vi "tvac_gui_chamber_workingcopy.vi"() -> ()   [LabVIEW 2017]
uses:
  <vilib>/httpClient/ClientHandle.ctl
  msg7171_linux.llb/send single message.vi
  <vilib>/httpClient/POSTBuffer.vi
  <vilib>/httpClient/LabVIEWHTTPClient.lvlib
panel:
  in  "Read MCC":bool
  in  "Read Pressure Gauges":bool
  out "output cluster":T1
  out "Cluster":T2
  in  "Custom Graph Selector":i32
  in  "exit":bool
  in  "AlarmColor":u32(colorbox)
  in  "Alarm String":string
  in  "Plot Color":u32(colorbox)=16860
  in  "Temperature":dbl format="%#_13g"
  in  "TC Label":string
  in  "Graph ON/OFF":u32(colorbox)=4250624
  in  "index (col)":i32
  in  "index (row)":i32
  out "working array":bool[](array[boolean])
  in  "Local Debug":bool
  in  "Tab Control":enum32{"TCs", "Graphs", "Thermal Profile"}(tab)
  in  "Log/Linear Y-Axis":u16(ring) items=["Linear", "Log"]
  in  "Total Time":dbl
  in  "Set Time TC Graph":bool
  in  "Graphing Selection":u16(ring) items=["User Selection", "Graph All Thermocouples", "Clear Graph"]
  in  "Time Scale":u16(ring) items=["Minutes", "Hours", "Seconds"]
  out "Waveform Chart":waveform(dbl)[](graph)
  out "Thermocouples":T3(array[cluster])
  in  "Log/Linear Y-Axis 6":u16(ring) items=["Linear", "Log"]
  in  "Log/Linear Y-Axis 5":u16(ring) items=["Linear", "Log"]
  in  "Log/Linear Y-Axis 3":u16(ring) items=["Linear", "Log"]
  in  "Log/Linear Y-Axis 2":u16(ring) items=["Linear", "Log"]
  in  "Total Time 6":dbl
  in  "Set Time TC Graph 6":bool
  in  "Time Scale 6":u16(ring) items=["Minutes", "Hours", "Seconds"]
  in  "Total Time 5":dbl
  in  "Set Time TC Graph 5":bool
  in  "Time Scale 5":u16(ring) items=["Minutes", "Hours", "Seconds"]
  in  "Total Time 4":dbl
  in  "Set Time TC Graph 4":bool
  in  "Time Scale 4":u16(ring) items=["Minutes", "Hours", "Seconds"]
  in  "Total Time 3":dbl
  in  "Set Time TC Graph 3":bool
  in  "Time Scale 3":u16(ring) items=["Minutes", "Hours", "Seconds"]
  in  "Total Time 2":dbl
  in  "Set Time TC Graph 2":bool
  in  "Time Scale 2":u16(ring) items=["Minutes", "Hours", "Seconds"]
  in  "Log/Linear Y-Axis 1":u16(ring) items=["Linear", "Log"]
  in  "Total Time 1":dbl
  in  "Set Time TC Graph 1":bool
  in  "Time Scale 1":u16(ring) items=["Minutes", "Hours", "Seconds"]
  in  "Custom Chart 2 Selection":i32[](listbox)=[0]
  in  "Custom Chart 1 Selection":i32[](listbox)=[0]
  out "Custom Chart 1":waveform(dbl)[](graph)
  in  "Custom Chart 3 Selection":i32[](listbox)=[0]
  in  "Custom Chart 4 Selection":i32[](listbox)=[0]
  in  "Custom Chart 5 Selection":i32[](listbox)=[0]
  in  "Custom Chart 6 Selection":i32[](listbox)=[0]
  out "Custom Chart 2":waveform(dbl)[](graph)
  out "Custom Chart 3":waveform(dbl)[](graph)
  out "Custom Chart 4":waveform(dbl)[](graph)
  out "Custom Chart 5":waveform(dbl)[](graph)
  out "Custom Chart 6":waveform(dbl)[](graph)
  in  "Log/Linear Y-Axis 4":u16(ring) items=["Linear", "Log"]
  in  "Set Z 1":bool
  in  "Z3 Thermal Profile":i32(listbox)
  in  "Z2 Thermal Profile":i32(listbox)
  in  "Z1 Thermal Profile":i32(listbox)
  in  "Zone 3 Temp":u16(ring) items=["Average", "Minimum", "Maximum"]
  in  "Zone 2 Temp":u16(ring) items=["Average", "Minimum", "Maximum"]
  in  "Zone 1 Temp":u16(ring) items=["Average", "Minimum", "Maximum"]
  in  "Zone 1 TC":i32[](listbox)=[0]
  in  "Zone 2 TC":i32[](listbox)=[0]
  in  "Zone 3 TC":i32[](listbox)=[0]
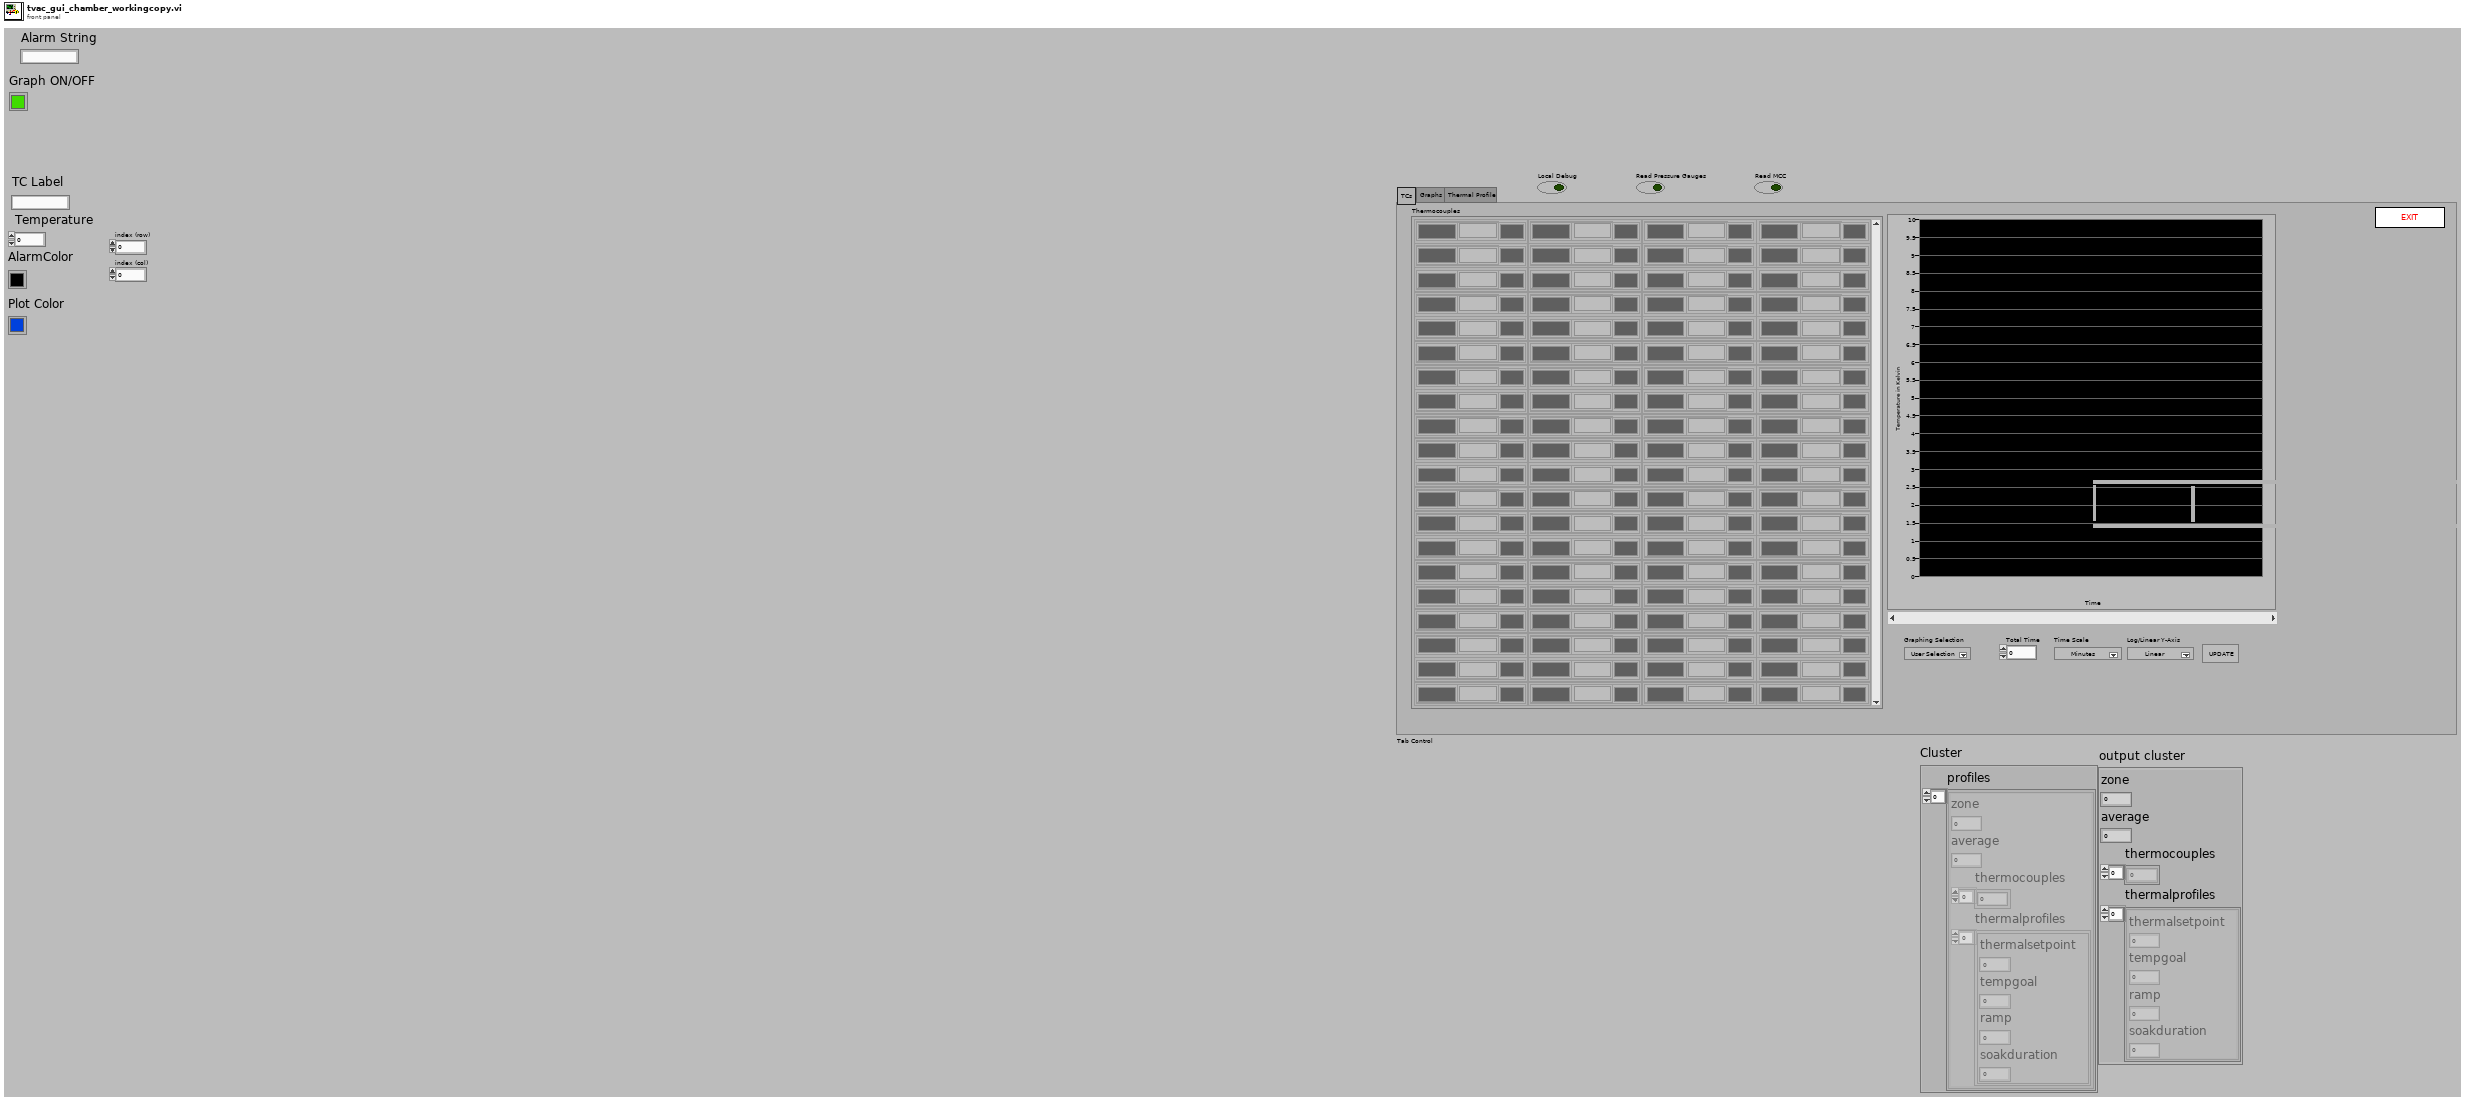
[diagram p1: front panel]
types:
  T1 = cluster{"zone":i32, "average":i32, "thermocouples":dbl[], "thermalprofiles":cluster{"thermalsetpoint":i32, "tempgoal":i32, "ramp":i32, "soakduration":i32}[]}
  T2 = cluster{"profiles":cluster{"zone":i32, "average":i32, "thermocouples":dbl[], "thermalprofiles":cluster{"thermalsetpoint":i32, "tempgoal":i32, "ramp":i32, "soakduration":i32}[]}[]}
  T3 = cluster{"TC Label":string, "Alarm Status":string, "Alarm Color":u32, "Temperature":string, "PlotColor":u32, "Graph On/Off":u32}[][]
  T4 = cluster{"Cp Stage 1 Temp":dbl[], "Cp Stage 2 Temp":dbl[], "Compressor Temp":dbl[]}
  T5 = typedef "LabVIEWHTTPClient.lvlib/ClientHandle.ctl" = refnum<k1>
  T6 = cluster{"go":bool, "Http session":T5, "URL prefex":string, "index (row)":i32, "index (col)":i32, "Graph ON/OFF":u32, "TC Label":string, "Temperature":dbl, "AlarmColor":u32, "Plot Color":u32, "Alarm String":string, "Thermocouples":cluster{"TC Label":string, "Alarm Status":string, "Alarm Color":u32, "Temperature":string, "PlotColor":u32, "Graph On/Off":u32}[][], "working array":bool[], "i":i32, "NumberTCs":i32, "Waveform Chart":waveform(dbl)[], "Custom Chart 1":waveform(dbl)[], "Pressure":dbl[], "numSensors":i32, "Database":dbl[], "PumpTemps":cluster{"Cp Stage 1 Temp":dbl[], "Cp Stage 2 Temp":dbl[], "Compressor Temp":dbl[]}, "Zones":dbl[]}
  T7 = cluster{"TC Label":string, "Alarm Status":string, "Alarm Color":u32, "Temperature":string, "PlotColor":u32, "Graph On/Off":u32}
  T8 = cluster{"Cryopump Stage 1 Temp":dbl[], "Cryopump Stage 2 Temp":dbl[], "Compressor Temp":dbl[]}
  T9 = cluster{"DutyCycle":i32, "Stage1Temp":i32, "CryoPumpReadyState":cluster{"MotorOn":bool, "Ready":bool}, "PurgeValveState":bool, "RegenError":string, "RegenStep":string, "RoughingValveState":bool, "RoughingInterlock":cluster{"RoughingPermission":bool, "RoughingNeeded":bool, "Cryopumprunning":bool}, "Stage2Temp":i32, "Status":cluster{"PumpOn":bool, "RoughOpen":bool, "PurgeOpen":bool, "ThermocoupleGaugeOn":bool, "PowerFailureOccurred":bool}, "TcPressure":i32}
  T10 = cluster{"time":string, "TCs":cluster{"thermocouple":i32, "time":dbl, "temp":dbl, "working":bool, "alarm":i32}[]}
  T11 = cluster{"thermocouple":i32, "time":dbl, "temp":dbl, "working":bool, "alarm":i32}[]
  T12 = typedef "LVPositionTypeDef.ctl" = cluster{"Left":i32, "Top":i32}
  T13 = typedef "LVPoint32TypeDef.ctl" = cluster{"Horizontal":i32, "Vertical":i32}
  T14 = typedef "LVRangeTypeDef.ctl" = cluster{"Minimum":dbl, "Maximum":dbl, "Increment":dbl, "Minor Increment":dbl, "Start":dbl}
  T15 = cluster{"Pressure[0]":dbl, "Pressure[1]":dbl, "Pressure[2]":dbl}
  T16 = cluster{"zone":i32, "average":i32, "thermocouples":dbl[], "thermalprofiles":cluster{"thermalsetpoint":i32, "tempgoal":i32, "ramp":i32, "soakduration":i32}[]}[]
  T17 = cluster{"profiles[0]":cluster{"zone":i32, "average":i32, "thermocouples":dbl[], "thermalprofiles":cluster{"thermalsetpoint":i32, "tempgoal":i32, "ramp":i32, "soakduration":i32}[]}, "profiles[1]":cluster{"zone":i32, "average":i32, "thermocouples":dbl[], "thermalprofiles":cluster{"thermalsetpoint":i32, "tempgoal":i32, "ramp":i32, "soakduration":i32}[]}, "profiles[2]":cluster{"zone":i32, "average":i32, "thermocouples":dbl[], "thermalprofiles":cluster{"thermalsetpoint":i32, "tempgoal":i32, "ramp":i32, "soakduration":i32}[]}, "profiles[3]":cluster{"zone":i32, "average":i32, "thermocouples":dbl[], "thermalprofiles":cluster{"thermalsetpoint":i32, "tempgoal":i32, "ramp":i32, "soakduration":i32}[]}, "profiles[4]":cluster{"zone":i32, "average":i32, "thermocouples":dbl[], "thermalprofiles":cluster{"thermalsetpoint":i32, "tempgoal":i32, "ramp":i32, "soakduration":i32}[]}, "profiles[5]":cluster{"zone":i32, "average":i32, "thermocouples":dbl[], "thermalprofiles":cluster{"thermalsetpoint":i32, "tempgoal":i32, "ramp":i32, "soakduration":i32}[]}, "profiles[6]":cluster{"zone":i32, "average":i32, "thermocouples":dbl[], "thermalprofiles":cluster{"thermalsetpoint":i32, "tempgoal":i32, "ramp":i32, "soakduration":i32}[]}, "profiles[7]":cluster{"zone":i32, "average":i32, "thermocouples":dbl[], "thermalprofiles":cluster{"thermalsetpoint":i32, "tempgoal":i32, "ramp":i32, "soakduration":i32}[]}, "profiles[8]":cluster{"zone":i32, "average":i32, "thermocouples":dbl[], "thermalprofiles":cluster{"thermalsetpoint":i32, "tempgoal":i32, "ramp":i32, "soakduration":i32}[]}}
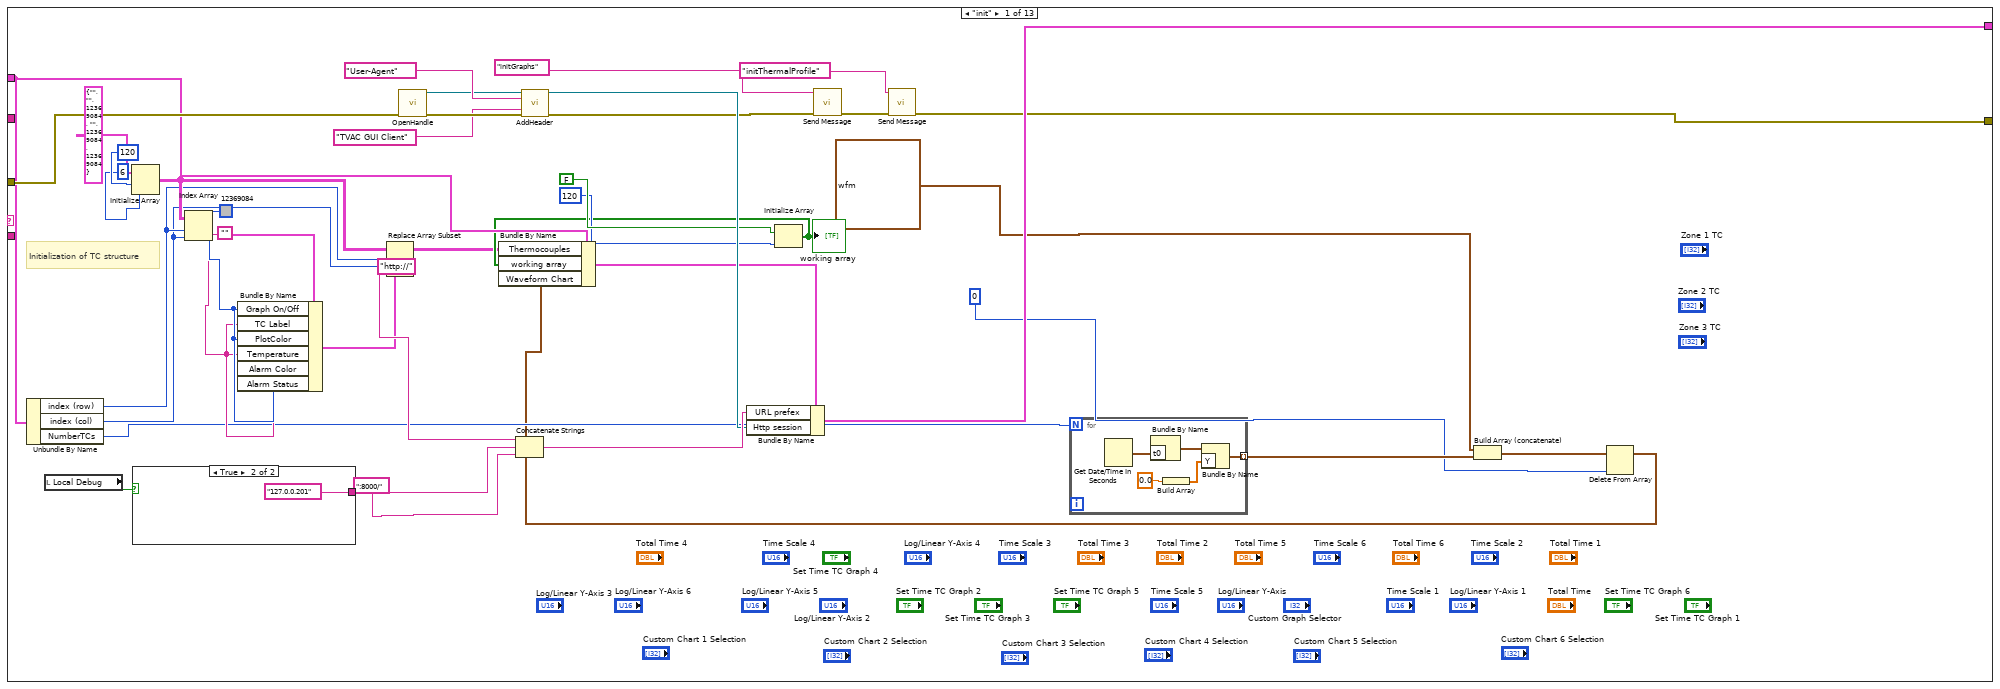
[diagram p2: hidden frame]
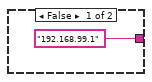
[diagram p3: hidden frame]
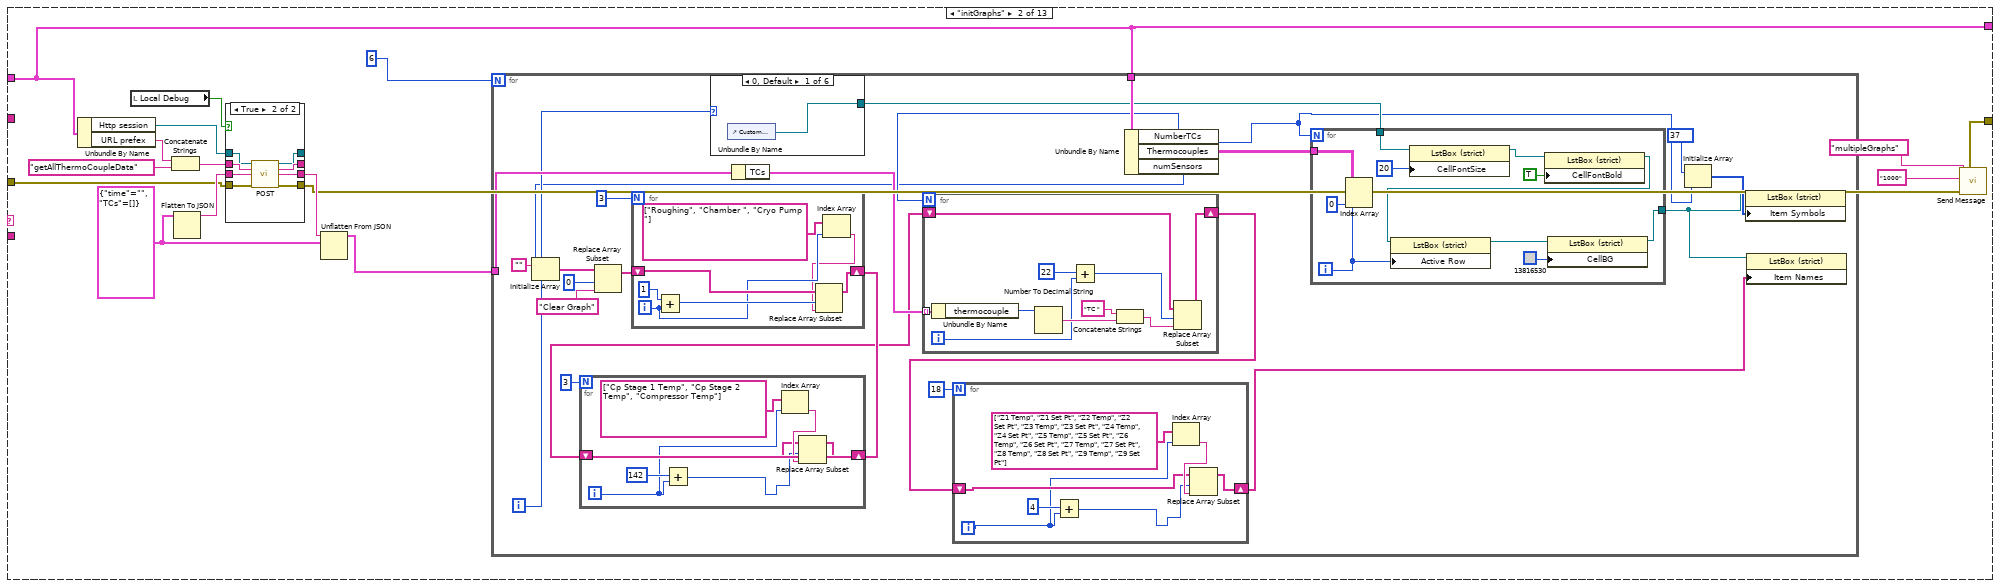
[diagram p4: hidden frame]
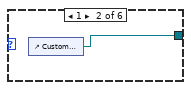
[diagram p5: hidden frame]
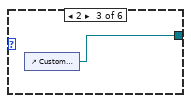
[diagram p6: hidden frame]
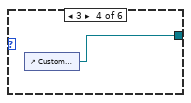
[diagram p7: hidden frame]
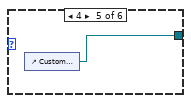
[diagram p8: hidden frame]
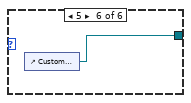
[diagram p9: hidden frame]
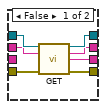
[diagram p10: hidden frame]
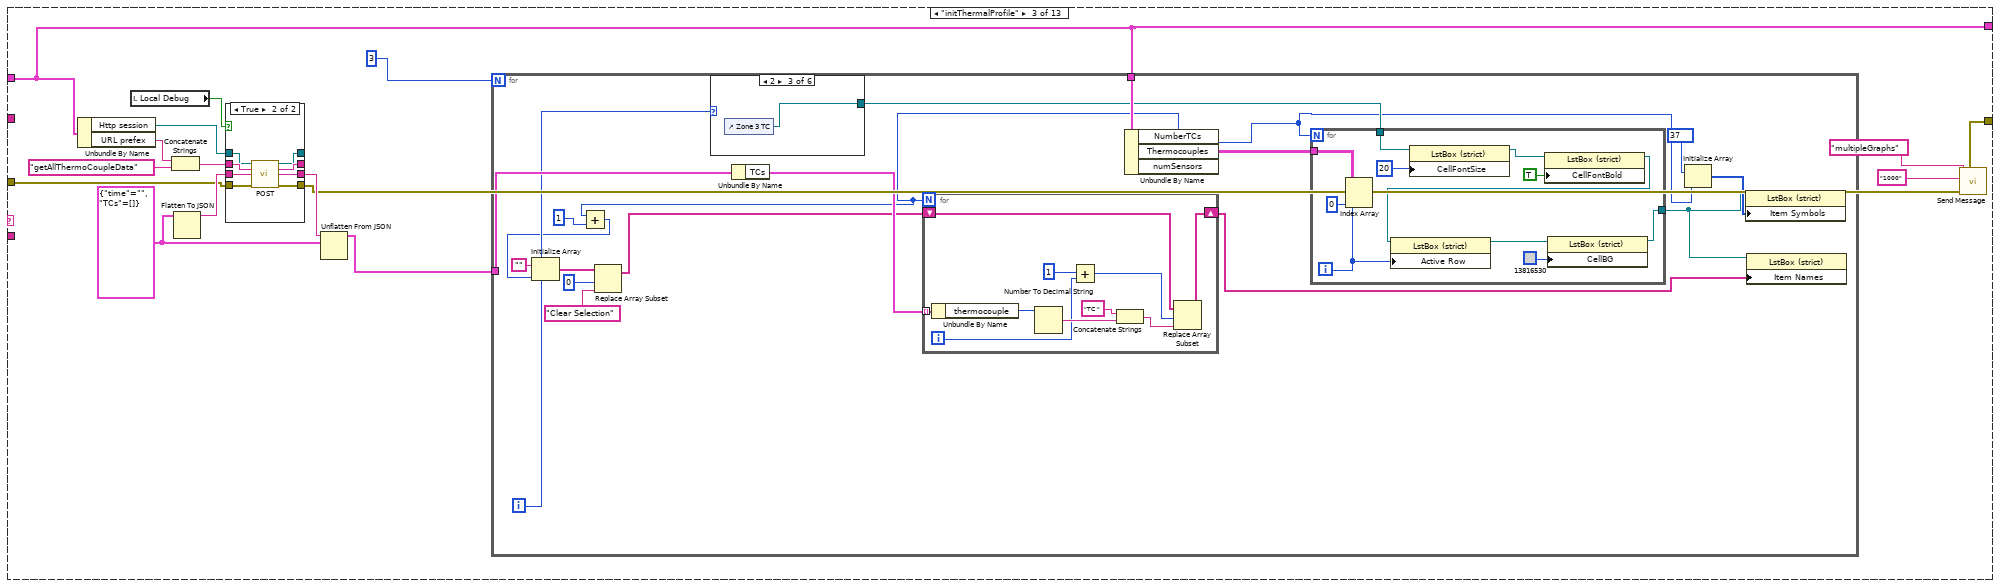
[diagram p11: hidden frame]
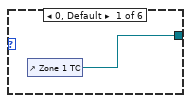
[diagram p12: hidden frame]
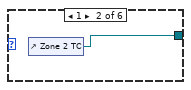
[diagram p13: hidden frame]
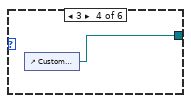
[diagram p14: hidden frame]
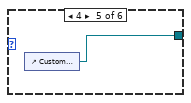
[diagram p15: hidden frame]
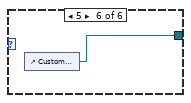
[diagram p16: hidden frame]
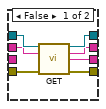
[diagram p17: hidden frame]
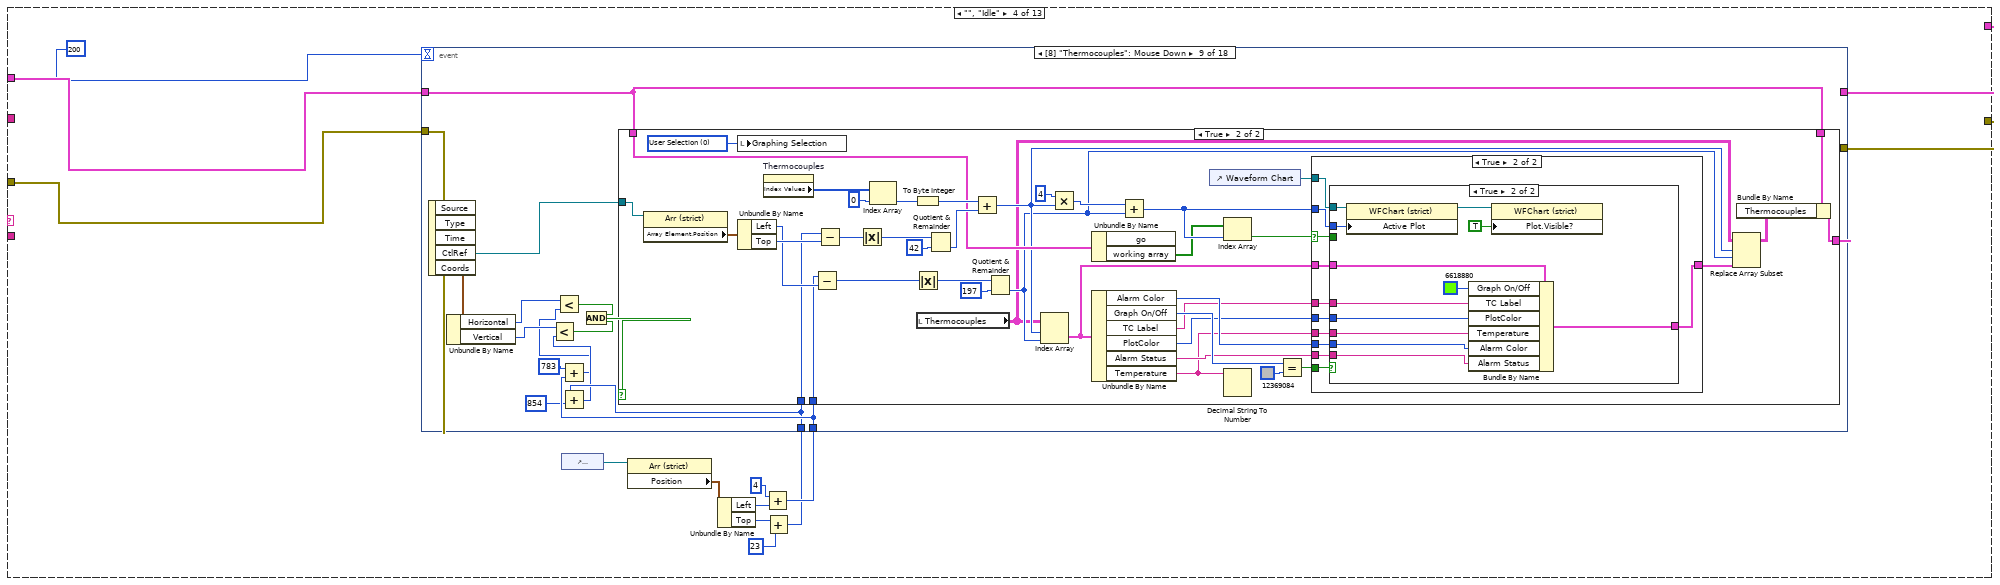
[diagram p18: hidden frame]
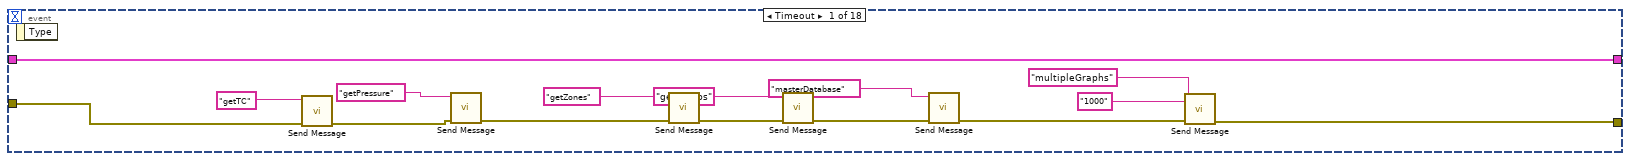
[diagram p19: hidden frame]
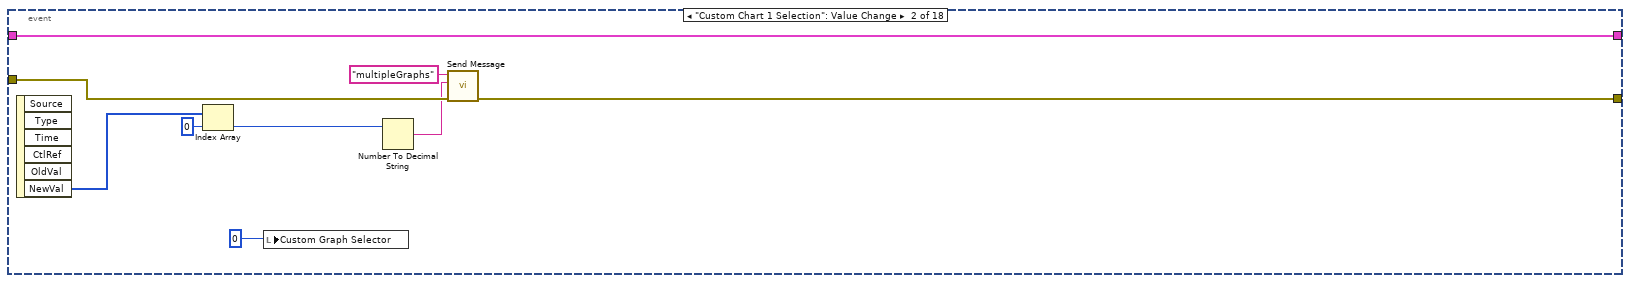
[diagram p20: hidden frame]
diagram:
  w2 = T4 {"Cp Stage 1 Temp"=[0.0], "Cp Stage 2 Temp"=[0.0], "Compressor Temp"=[0.0]}  # PumpTemps
  w5 = dbl[] []  # Pressure
  w25 = ""  # URL prefex
  w26 = T5 refnum  # Http session
  w27 = TRUE  # go
  n1 = call "Register Module.vi"() -> ("error out"=w23:errorcluster)  [unwired: 10 in, 1 out]
  n2 = call-poly "Send Message.vi"("error in (no error)"=w23, "event"="init") -> ("error out"=w22:errorcluster)  [unwired: 9 in]
  n3 = local read "Waveform Chart"() -> (w9:waveform(dbl)[])
  n4 = local read "Thermocouples"() -> (w7:T3)
  n5 = local read "Custom Chart 1"() -> (w6:waveform(dbl)[])
  n6 = Bundle("go"=w27, "Http session"=w26, "URL prefex"=w25, "index (row)"="index (row)", "index (col)"="index (col)", "Graph ON/OFF"="Graph ON/OFF", "TC Label"="TC Label", "Temperature"="Temperature", "AlarmColor"="AlarmColor", "Plot Color"="Plot Color", "Alarm String"="Alarm String", "Thermocouples"=w7, "working array"=bool[] [TRUE, TRUE, TRUE, TRUE, TRUE, TRUE, TRUE, TRUE, TRUE, TRUE, TRUE, TRUE, TRUE, TRUE, TRUE, TRUE, TRUE, TRUE, TRUE, TRUE, TRUE, TRUE, TRUE, TRUE, TRUE, TRUE, TRUE, TRUE, TRUE, TRUE, TRUE, TRUE, TRUE, TRUE, TRUE, TRUE, TRUE, TRUE, TRUE, TRUE, TRUE, TRUE, TRUE, TRUE, TRUE, TRUE, TRUE, TRUE, TRUE, TRUE, TRUE, TRUE, TRUE, TRUE, TRUE, TRUE, TRUE, TRUE, TRUE, TRUE, TRUE, TRUE, TRUE, TRUE, TRUE, TRUE, TRUE, TRUE, TRUE, TRUE, TRUE, TRUE, TRUE, TRUE, TRUE, TRUE, TRUE, TRUE, TRUE, TRUE, TRUE, TRUE, TRUE, TRUE, TRUE, TRUE, TRUE, TRUE, TRUE, TRUE, TRUE, TRUE, TRUE, TRUE, TRUE, TRUE, TRUE, TRUE, TRUE, TRUE, TRUE, TRUE, TRUE, TRUE, TRUE, TRUE, TRUE, TRUE, TRUE, TRUE, TRUE, TRUE, TRUE, TRUE, TRUE, TRUE, TRUE, TRUE, TRUE, TRUE], "i"=0, "NumberTCs"=120, "Waveform Chart"=w9, "Custom Chart 1"=w6, "Pressure"=w5, "numSensors"=145, "Database"=dbl[] [0.0, 1000.5841582194602, 1000.5841582194602, 1000.5841582194602, 0.6389895835935778, 0.7578061575842531, 1.153531014677555, 1.4572061556343079, 1.0192558642672256, 0.9245021790184325, 0.34311035179988925, 1.1970333160202968, 1.066989851322369, 0.5926593131154867, 0.7219240511326698, 1.0529790116491695, 1.4485694746891444, 0.9139060201605569, 0.7997359753068659, 0.6568795179977746, 0.8470104541419833, 1.0272585161866683, 0.6577301535824354, 0.645139941938139, 1.5235316442408067, 0.5128651184775285, 1.6421980587090137, 1.3961508335147417, 1.1242639015795428, 1.5954313466624428, 1.1919135255187876, 1.2615004458206727, 1.1320092264321664, 1.922759836270222, 1.1315561200367314, 1.4924621723754858, 0.6988771274186227, 1.069709701591943, 0.9920698240997152, 0.5395549253287656, 0.42891479657680576, 1.2794224940227927, 0.2687949632437338, 0.16127136772755854, 1.0174597006256374, 1.2079238230365172, 0.9745554383837218, 1.5348516925460962, 0.9488878852839246, 1.6634477658652282, 1.1924291951744272, 1.2231949298067308, 1.2223766746774598, 1.30664154589907, 1.2872878364107239, 0.5274250065177812, 0.7905999067114673, 1.2748974665085449, 1.216972941585413, 0.959115576325391, 0.5743502840762814, 0.8219540421676025, 0.613053899308251, 1.3785560870413707, 1.034117232127813, 1.1237698659753859, 1.4495548642149667, 0.6967905980938514, 0.6224497255665377, 1.6551326273040576, 1.2103048396824558, 0.6078721016951973, 1.3790669246280296, 0.5454332940871525, 1.5318777012492035, 1.2496539590411258, 0.9145395304446965, 1.3855381787793546, 1.0857600342029163, 1.3185833631438346, 0.9769688683142593, 1.026663691242448, 0.6744610422623843, 1.1965175398567691, 0.4847084945450119, 0.6435799980029115, 0.8079659363810663, 0.9130053929540112, 0.5271098423006861, 0.8088111736464799, 1.1455315536576556, 1.139809531926708, 1.5840192673434794, 1.0296748968089129, 1.7370669751200136, 1.3715484550405317, 0.3362063953932494, 1.0385868418202253, 1.4947740276021626, 1.0393600693910505, 0.8870410800672984, 1.2470388696569872, 0.9846724980375481, 0.9952471377109308, 1.0807485178906029, 1.1016630607035562, 1.3301039036808464, 0.8856852816151205, 0.4719509873120426, 0.5191430277856135, 0.12135113366044793, 0.4230478635224125, 1.1140562049976255, 1.5484968368781251, 1.1999891199114734, 1.8721302183420216, 1.071489235222563, 0.6260864330445979, 1.0305668002030492, 1.0223711899566386, 0.7842533472819472, 1.7301290335750898, 1.318694748426881, 0.6978662965493679], "PumpTemps"=w2, "Zones"=dbl[] [24.54828257301887, 25.0, 20.035959453954195, 26.0, 28.926820041278148, 27.0, 21.321976066931608, 28.0, 29.197600688359813, 29.0, 29.117373424110085, 30.0, 21.092914485312942, 31.0, 27.791581465649088, 32.0, 24.70861457288988, 33.0]) -> (w13:T6)  [unwired: 1 in]
  n7 = while {
    shift-left: w13 -> [w32]
    shift-right: [w29] -> _
    shift-right: [w30] -> w8
    shift-left: w22 -> [w37]
    stop <- w28 continue-if-true
    n8 = call "Get Message.vi"("error in (no error)"=w37) -> ("error out"=w35:errorcluster, "event buffer"=w36:string, "event"=w34:string, "source"=w33:string)  [unwired: 7 in]
    n9 = case shown="\"getZones\"" w34 {
      selector: w34 -> [_ _ _ _ _ _ _ _ _ _ _ _ w1352]
      tunnel: [w69 w90 w192 w273 w947 w984 w1099 w1139 w1184 w1204 w1335 w1350 w1354] -> w29
      tunnel: w32 -> [w50 w90 w192 w275 w950 w990 w1094 w1134 w1185 w1204 w1335 w1346 w1354]
      tunnel: w36 -> [_ _ _ _ _ _ _ _ _ w1205 _ _ _]
      tunnel: w35 -> [w72 w89 w191 w274 w949 w1006 w1093 w1140 w1190 _ _ w1349 w1353]
      tunnel: [w39 w85 w187 w272 w948 w980 w1093 w1140 w1190 _ _ w1348 w1351] -> w31
      tunnel: w33 -> [_ _ _ _ _ _ _ _ _ _ _ _ _]
      frame "init" {
        w55 = ""
        w56 = u32 12369084 ("PlotColor")
        # "Initialization of TC structure"
        n10 = Unbundle By Name(w50) -> ("index (row)"=w58:i32, "index (col)"=w57:i32, "NumberTCs"=w47:i32)
        n11 = local read "Local Debug"() -> (w63:bool)
        n12 = Initialize Array(T7 {"TC Label"="", "Alarm Status"="", "Alarm Color"=12369084, "Temperature"="", "PlotColor"=12369084, "Graph On/Off"=12369084}, 120 ("dimension size"), 6 ("dimension size")) -> (w59:T3)
        n13 = case shown="True" w63 {
          tunnel: ["192.168.99.1" ("Address") "127.0.0.201" ("Address")] -> w64
          frame False {
          }
          frame True {
          }
        }
        n14 = Index Array(array=w59, index (row)=w58, index (col)=w57) -> (element=w54:T7)
        n15 = Bundle By Name(cluster=w54, "Graph On/Off"=w56, "TC Label"=w55, "PlotColor"=w56, "Temperature"=w55, "Alarm Color"=w56, "Alarm Status"=w55) -> (w53:T7)
        n16 = Replace Array Subset(array=w59, new element=w53, index (row)=w58, index (col)=w57) -> (w41:T3)
        n17 = call <vilib>:"OpenHandle.vi"("error in (no error)"=w72) -> ("client handle out"=w73:T5, "error out"=w76:errorcluster)  [unwired: 13 in]
        n18 = Concatenate Strings("http://" ("url"), w64, ":8000/" ("url")) -> (w68:string)
        n19 = call <vilib>:"AddHeader.vi"("client handle"=w73, "header"="User-Agent", "value"="TVAC GUI Client", "error in (no error)"=w76) -> ("client handle out"=w67:T5, "error out"=w66:errorcluster)  [unwired: 10 in]
        n20 = Initialize Array(FALSE ("Boolean"), 120 ("dimension size")) -> (w48:bool[])
        "working array" <- w48
        n21 = call-poly "Send Message.vi"("error in (no error)"=w66, "event"="initGraphs") -> ("error out"=w40:errorcluster)  [unwired: 9 in]
        n22 = call-poly "Send Message.vi"("error in (no error)"=w40, "event"="initThermalProfile") -> ("error out"=w39:errorcluster)  [unwired: 9 in]
        n23 = for {
          N: w47 -> [_]
          tunnel: [w77] -> w45 mode=indexing
          n24 = Get Date/Time In Seconds() -> (seconds since 1Jan1904=w81:timestamp)
          n25 = Bundle By Name("t0"=w81) -> (w78:waveform(dbl))  [unwired: 1 in]
          n26 = Build Array(0.0) -> (w80:dbl[])
          n27 = Bundle By Name(cluster=w78, "Y"=w80) -> (w77:waveform(dbl))
        }
        n28 = Build Array (concatenate)(waveform(dbl) {"t0"=timestamp(0 s since 1904-01-01), "dt"=1.0, "Y"=[0.0]} ("element"), w45) -> (w46:waveform(dbl)[])
        n29 = Delete From Array(array=w46, index=0) -> (array with subset deleted=w44:waveform(dbl)[])  [unwired: 1 in, 1 out]
        n30 = Bundle By Name(cluster=w50, "Thermocouples"=w41, "working array"=w48, "Waveform Chart"=w44) -> (w49:T6)
        n31 = Bundle By Name(cluster=w49, "URL prefex"=w68, "Http session"=w67) -> (w69:T6)
      }
      frame "initGraphs" {
        w93 = T10 {"time"="", "TCs"=[]} ("Cluster")
        n32 = Unbundle By Name(w90) -> ("Http session"=w99:T5, "URL prefex"=w97:string)
        n33 = local read "Local Debug"() -> (w91:bool)
        n34 = Concatenate Strings(w97, "getAllThermoCoupleData" ("url")) -> (w98:string)
        n35 = Flatten To JSON(anything=w93) -> (JSON string=w92:string)  [unwired: 2 in, 1 out]
        n36 = case shown="True" w91 {
          tunnel: w89 -> [w177 w178]
          tunnel: [w176 w179] -> w86
          tunnel: [w175 w180] -> _
          tunnel: w99 -> [w174 w183]
          tunnel: w98 -> [w173 w184]
          tunnel: [w172 w181] -> w95
          tunnel: [w171 w182] -> _
          tunnel: w92 -> [_ w185]
          frame False {
            n37 = call <vilib>:"GET.vi"("client handle"=w174, "url"=w173, "error in (no error)"=w177) -> ("client handle out"=w175:T5, "headers"=w171:string, "body"=w172:string, "error out"=w176:errorcluster)  [unwired: 9 in]
          }
          frame True {
            n38 = call-poly <vilib>:"POST.vi"("client handle"=w183, "url"=w184, "buffer"=w185, "error in (no error)"=w178) -> ("client handle out"=w180:T5, "headers"=w182:string, "body"=w181:string, "error out"=w179:errorcluster)  [unwired: 8 in]
          }
        }
        n39 = Unflatten From JSON(JSON string=w95, type and defaults=w93) -> (value=w94:T10)  [unwired: 5 in, 1 out]
        n40 = for {
          N: 6 ("Numeric") -> [_]
          tunnel: w94 -> [w121]
          tunnel: w90 -> [w120]
          i -> [w103]
          n41 = case shown="0, Default" w103 {
            tunnel: [w123 w124 w125 w126 w127 w128] -> w104
            frame 0, Default {
              n42 = control-ref of="Custom Chart 1 Selection"() -> (w123:refnum<vi>)
            }
            frame 1 {
              n43 = control-ref of="Custom Chart 2 Selection"() -> (w124:refnum<vi>)
            }
            frame 2 {
              n44 = control-ref of="Custom Chart 3 Selection"() -> (w125:refnum<vi>)
            }
            frame 3 {
              n45 = control-ref of="Custom Chart 4 Selection"() -> (w126:refnum<vi>)
            }
            frame 4 {
              n46 = control-ref of="Custom Chart 5 Selection"() -> (w127:refnum<vi>)
            }
            frame 5 {
              n47 = control-ref of="Custom Chart 6 Selection"() -> (w128:refnum<vi>)
            }
          }
          n48 = Unbundle By Name(w121) -> ("TCs"=w117:T11)
          n49 = Unbundle By Name(w120) -> ("NumberTCs"=w115:i32, "Thermocouples"=w122:T3, "numSensors"=w101:i32)
          n50 = Initialize Array("", w101) -> (w113:string[])
          n51 = Replace Array Subset(array=w113, new element="Clear Graph" ("new element/subarray"), index=0) -> (w110:string[])
          n52 = for {
            N: 3 -> [_]
            shift-right: [w148] -> w108
            shift-left: w110 -> [w149]
            i -> [w144]
            n53 = Add(x=1 ("index"), y=w144) -> (x+y=w146:i32)
            n54 = Index Array(array=string[] ["Roughing", "Chamber ", "Cryo Pump "], index=w144) -> (element=w143:string)
            n55 = Replace Array Subset(array=w149, new element=w143, index=w146) -> (w148:string[])
          }
          n56 = for {
            N: 3 -> [_]
            shift-right: [w139] -> w107
            shift-left: w108 -> [w140]
            i -> [w136]
            n57 = Add(x=142 ("index"), y=w136) -> (x+y=w137:i32)
            n58 = Index Array(array=string[] ["Cp Stage 1 Temp", "Cp Stage 2 Temp", "Compressor Temp"], index=w136) -> (element=w141:string)
            n59 = Replace Array Subset(array=w140, new element=w141, index=w137) -> (w139:string[])
          }
          n60 = for {
            N: w115 -> [_]
            tunnel: w117 -> [w156] mode=indexing
            shift-right: [w150] -> w100
            shift-left: w107 -> [w152]
            i -> [w154]
            n61 = Unbundle By Name(w156) -> ("thermocouple"=w157:i32)
            n62 = Number To Decimal String(number=w157) -> (decimal integer string=w159:string)  [unwired: 1 in]
            n63 = Add(x=22 ("index"), y=w154) -> (x+y=w153:i32)
            n64 = Concatenate Strings("TC " ("string"), w159) -> (w151:string)
            n65 = Replace Array Subset(array=w152, new element=w151, index=w153) -> (w150:string[])
          }
          n66 = for {
            N: 18 -> [_]
            shift-right: [w129] -> w106
            shift-left: w100 -> [w131]
            i -> [w130]
            n67 = Add(x=4 ("index"), y=w130) -> (x+y=w132:i32)
            n68 = Index Array(array=string[] ["Z1 Temp", "Z1 Set Pt", "Z2 Temp", "Z2 Set Pt", "Z3 Temp", "Z3 Set Pt", "Z4 Temp", "Z4 Set Pt", "Z5 Temp", "Z5 Set Pt", "Z6 Temp", "Z6 Set Pt", "Z7 Temp", "Z7 Set Pt", "Z8 Temp", "Z8 Set Pt", "Z9 Temp", "Z9 Set Pt"], index=w130) -> (element=w134:string)
            n69 = Replace Array Subset(array=w131, new element=w134, index=w132) -> (w129:string[])
          }
          n70 = for {
            N: w101 -> [_]
            tunnel: w122 -> [w170]
            tunnel: w104 -> [w164]
            tunnel: [w160] -> w102
            i -> [w167]
            n71 = Index Array(array=w170, index (row)=w167, index (col)=0 ("disabled index (col)")) -> ()  [unwired: 1 out]
            n72 = property on="Property Node" class="LstBox (strict)"(reference=w164, "CellFontSize"=u32 20 ("Active Row:Cell Font:Size")) -> (reference out=w163:refnum<vi>)  [unwired: 1 in, 1 out]
            n73 = property on="Property Node" class="LstBox (strict)"(reference=w163, "CellFontBold"=TRUE ("Active Row:Cell Font:Bold")) -> (reference out=w162:refnum<vi>)  [unwired: 1 in, 1 out]
            n74 = property on="Property Node" class="LstBox (strict)"(reference=w162, "Active Row"=w167) -> (reference out=w161:refnum<vi>)  [unwired: 1 in, 1 out]
            n75 = property on="Property Node" class="LstBox (strict)"(reference=w161, "CellBG"=u32 13816530 ("Active Row:Cell Background Color")) -> (reference out=w160:refnum<vi>)  [unwired: 1 in, 1 out]
          }
          n76 = Initialize Array(37, w101) -> (w118:i32[])
          n77 = property on="Property Node" class="LstBox (strict)"(reference=w102, "Item Symbols"=w118) -> ()  [unwired: 1 in, 2 out]
          n78 = property on="Property Node" class="LstBox (strict)"(reference=w102, "Item Names"=w106) -> ()  [unwired: 1 in, 2 out]
        }
        n79 = call-poly "Send Message.vi"("error in (no error)"=w86, "event buffer"="1000", "event"="multipleGraphs") -> ("error out"=w85:errorcluster)  [unwired: 8 in]
      }
      frame "initThermalProfile" {
        w195 = T10 {"time"="", "TCs"=[]} ("Cluster")
        n80 = Unbundle By Name(w192) -> ("Http session"=w201:T5, "URL prefex"=w199:string)
        n81 = local read "Local Debug"() -> (w193:bool)
        n82 = Concatenate Strings(w199, "getAllThermoCoupleData" ("url")) -> (w200:string)
        n83 = Flatten To JSON(anything=w195) -> (JSON string=w194:string)  [unwired: 2 in, 1 out]
        n84 = case shown="True" w193 {
          tunnel: w191 -> [w254 w255]
          tunnel: [w253 w256] -> w188
          tunnel: [w252 w257] -> _
          tunnel: w201 -> [w251 w260]
          tunnel: w200 -> [w250 w261]
          tunnel: [w249 w258] -> w197
          tunnel: [w248 w259] -> _
          tunnel: w194 -> [_ w262]
          frame False {
            n85 = call <vilib>:"GET.vi"("client handle"=w251, "url"=w250, "error in (no error)"=w254) -> ("client handle out"=w252:T5, "headers"=w248:string, "body"=w249:string, "error out"=w253:errorcluster)  [unwired: 9 in]
          }
          frame True {
            n86 = call-poly <vilib>:"POST.vi"("client handle"=w260, "url"=w261, "buffer"=w262, "error in (no error)"=w255) -> ("client handle out"=w257:T5, "headers"=w259:string, "body"=w258:string, "error out"=w256:errorcluster)  [unwired: 8 in]
          }
        }
        n87 = Unflatten From JSON(JSON string=w197, type and defaults=w195) -> (value=w196:T10)  [unwired: 5 in, 1 out]
        n88 = for {
          N: 3 ("Numeric") -> [_]
          tunnel: w196 -> [w219]
          tunnel: w192 -> [w218]
          i -> [w209]
          n89 = case shown="2" w209 {
            tunnel: [w221 w222 w223 w224 w225 w226] -> w210
            frame 0, Default {
              n90 = control-ref of="Zone 1 TC"() -> (w221:refnum<vi>)
            }
            frame 1 {
              n91 = control-ref of="Zone 2 TC"() -> (w222:refnum<vi>)
            }
            frame 2 {
              n92 = control-ref of="Zone 3 TC"() -> (w223:refnum<vi>)
            }
            frame 3 {
              n93 = control-ref of="Custom Chart 4 Selection"() -> (w224:refnum<vi>)
            }
            frame 4 {
              n94 = control-ref of="Custom Chart 5 Selection"() -> (w225:refnum<vi>)
            }
            frame 5 {
              n95 = control-ref of="Custom Chart 6 Selection"() -> (w226:refnum<vi>)
            }
          }
          n96 = Unbundle By Name(w219) -> ("TCs"=w215:T11)
          n97 = Unbundle By Name(w218) -> ("NumberTCs"=w204:i32, "Thermocouples"=w220:T3, "numSensors"=w207:i32)
          n98 = Add(x=w204, y=1 ("index")) -> (x+y=w202:i32)
          n99 = Initialize Array("", w202) -> (w213:string[])
          n100 = Replace Array Subset(array=w213, new element="Clear Selection" ("new element/subarray"), index=0) -> (w206:string[])
          n101 = for {
            N: w204 -> [_]
            tunnel: w215 -> [w233] mode=indexing
            shift-right: [w227] -> w205
            shift-left: w206 -> [w229]
            i -> [w231]
            n102 = Unbundle By Name(w233) -> ("thermocouple"=w234:i32)
            n103 = Number To Decimal String(number=w234) -> (decimal integer string=w236:string)  [unwired: 1 in]
            n104 = Add(x=1 ("index"), y=w231) -> (x+y=w230:i32)
            n105 = Concatenate Strings("TC " ("string"), w236) -> (w228:string)
            n106 = Replace Array Subset(array=w229, new element=w228, index=w230) -> (w227:string[])
          }
          n107 = for {
            N: w207 -> [_]
            tunnel: w220 -> [w247]
            tunnel: w210 -> [w241]
            tunnel: [w237] -> w208
            i -> [w244]
            n108 = Index Array(array=w247, index (row)=w244, index (col)=0 ("disabled index (col)")) -> ()  [unwired: 1 out]
            n109 = property on="Property Node" class="LstBox (strict)"(reference=w241, "CellFontSize"=u32 20 ("Active Row:Cell Font:Size")) -> (reference out=w240:refnum<vi>)  [unwired: 1 in, 1 out]
            n110 = property on="Property Node" class="LstBox (strict)"(reference=w240, "CellFontBold"=TRUE ("Active Row:Cell Font:Bold")) -> (reference out=w239:refnum<vi>)  [unwired: 1 in, 1 out]
            n111 = property on="Property Node" class="LstBox (strict)"(reference=w239, "Active Row"=w244) -> (reference out=w238:refnum<vi>)  [unwired: 1 in, 1 out]
            n112 = property on="Property Node" class="LstBox (strict)"(reference=w238, "CellBG"=u32 13816530 ("Active Row:Cell Background Color")) -> (reference out=w237:refnum<vi>)  [unwired: 1 in, 1 out]
          }
          n113 = Initialize Array(37, w207) -> (w216:i32[])
          n114 = property on="Property Node" class="LstBox (strict)"(reference=w208, "Item Symbols"=w216) -> ()  [unwired: 1 in, 2 out]
          n115 = property on="Property Node" class="LstBox (strict)"(reference=w208, "Item Names"=w205) -> ()  [unwired: 1 in, 2 out]
        }
        n116 = call-poly "Send Message.vi"("error in (no error)"=w188, "event buffer"="1000", "event"="multipleGraphs") -> ("error out"=w187:errorcluster)  [unwired: 8 in]
      }
      frame "", "Idle" {
        n117 = control-ref of="Thermocouples"() -> (w270:refnum<vi>)
        n118 = property on="Property Node" class="Arr (strict)"(reference=w270) -> ("Position"=w269:T12)  [unwired: 1 in, 2 out]
        n119 = Unbundle By Name(w269) -> ("Left"=w268:i32, "Top"=w266:i32)
        n120 = Add(x=4, y=w268) -> (x+y=w264:i32)
        n121 = Add(x=w266, y=23 ("x")) -> (x+y=w263:i32)
        n122 = event shown="[8] \"Thermocouples\": Mouse Down" {
          selector: _ -> [_ _ _ _ _ _ _ _ _ _ _ _ _ _ _ _ _ _]
          dyn-events: _ -> [_ _ _ _ _ _ _ _ _ _ _ _ _ _ _ _ _ _]
          timeout: 200 ("milliseconds to wait") -> [_ _ _ _ _ _ _ _ _ _ _ _ _ _ _ _ _ _]
          tunnel: w274 -> [w289 w296 w305 w314 w323 w332 w341 w346 w361 w454 w518 w579 w640 w701 w762 w823 w884 w943]
          tunnel: [w288 w295 w304 w313 w322 w331 w340 w345 w361 w454 w518 w579 w640 w701 w762 w823 w884 w941] -> w272
          tunnel: [w290 w297 w306 w315 w324 w333 w342 w350 w362 w448 w519 w580 w641 w702 w763 w824 w885 w944] -> w273
          tunnel: w275 -> [w290 w297 w306 w315 w324 w333 w342 w350 w363 w450 w519 w580 w641 w702 w763 w824 w885 w944]
          tunnel: w264 -> [_ _ _ _ _ _ _ _ w360 _ _ _ _ _ _ _ _ _]
          tunnel: w263 -> [_ _ _ _ _ _ _ _ w357 _ _ _ _ _ _ _ _ _]
          event Timeout {
            n123 = event-data() -> ()  [unwired: 1 in, 1 out]
            n124 = call-poly "Send Message.vi"("error in (no error)"=w289, "event"="getTC") -> ("error out"=w285:errorcluster)  [unwired: 9 in]
            n125 = call-poly "Send Message.vi"("error in (no error)"=w285, "event"="getPressure") -> ("error out"=w282:errorcluster)  [unwired: 9 in]
            n126 = call-poly "Send Message.vi"("error in (no error)"=w282, "event"="getZones") -> ("error out"=w280:errorcluster)  [unwired: 9 in]
            n127 = call-poly "Send Message.vi"("error in (no error)"=w280, "event"="getTemps") -> ("error out"=w277:errorcluster)  [unwired: 9 in]
            n128 = call-poly "Send Message.vi"("error in (no error)"=w277, "event"="masterDatabase") -> ("error out"=w276:errorcluster)  [unwired: 9 in]
            n129 = call-poly "Send Message.vi"("error in (no error)"=w276, "event buffer"="1000", "event"="multipleGraphs") -> ("error out"=w288:errorcluster)  [unwired: 8 in]
          }
          event "Custom Chart 1 Selection": Value Change {
            n130 = event-data() -> ("NewVal"=w298:i32[])  [unwired: 1 in, 5 out]
            n131 = Index Array(array=w298, index=0) -> (element=w292:i32)
            n132 = local write "Custom Graph Selector"(0) -> ()
            n133 = Number To Decimal String(number=w292) -> (decimal integer string=w293:string)  [unwired: 1 in]
            n134 = call-poly "Send Message.vi"("error in (no error)"=w296, "event buffer"=w293, "event"="multipleGraphs") -> ("error out"=w295:errorcluster)  [unwired: 8 in]
          }
          event "Custom Chart 2 Selection": Value Change {
            n135 = event-data() -> ("NewVal"=w307:i32[])  [unwired: 1 in, 5 out]
            n136 = Index Array(array=w307, index=0) -> (element=w301:i32)
            n137 = local write "Custom Graph Selector"(1) -> ()
            n138 = Number To Decimal String(number=w301) -> (decimal integer string=w302:string)  [unwired: 1 in]
            n139 = call-poly "Send Message.vi"("error in (no error)"=w305, "event buffer"=w302, "event"="multipleGraphs") -> ("error out"=w304:errorcluster)  [unwired: 8 in]
          }
          event "Custom Chart 3 Selection": Value Change {
            n140 = event-data() -> ("NewVal"=w316:i32[])  [unwired: 1 in, 5 out]
            n141 = Index Array(array=w316, index=0) -> (element=w310:i32)
            n142 = local write "Custom Graph Selector"(2) -> ()
            n143 = Number To Decimal String(number=w310) -> (decimal integer string=w311:string)  [unwired: 1 in]
            n144 = call-poly "Send Message.vi"("error in (no error)"=w314, "event buffer"=w311, "event"="multipleGraphs") -> ("error out"=w313:errorcluster)  [unwired: 8 in]
          }
          event "Custom Chart 4 Selection": Value Change {
            n145 = event-data() -> ("NewVal"=w325:i32[])  [unwired: 1 in, 5 out]
            n146 = Index Array(array=w325, index=0) -> (element=w319:i32)
            n147 = local write "Custom Graph Selector"(3) -> ()
            n148 = Number To Decimal String(number=w319) -> (decimal integer string=w320:string)  [unwired: 1 in]
            n149 = call-poly "Send Message.vi"("error in (no error)"=w323, "event buffer"=w320, "event"="multipleGraphs") -> ("error out"=w322:errorcluster)  [unwired: 8 in]
          }
          event "Custom Chart 5 Selection": Value Change {
            n150 = event-data() -> ("NewVal"=w334:i32[])  [unwired: 1 in, 5 out]
            n151 = Index Array(array=w334, index=0) -> (element=w328:i32)
            n152 = local write "Custom Graph Selector"(4) -> ()
            n153 = Number To Decimal String(number=w328) -> (decimal integer string=w329:string)  [unwired: 1 in]
            n154 = call-poly "Send Message.vi"("error in (no error)"=w332, "event buffer"=w329, "event"="multipleGraphs") -> ("error out"=w331:errorcluster)  [unwired: 8 in]
          }
          event "Custom Chart 6 Selection": Value Change {
            n155 = event-data() -> ("NewVal"=w343:i32[])  [unwired: 1 in, 5 out]
            n156 = Index Array(array=w343, index=0) -> (element=w337:i32)
            n157 = local write "Custom Graph Selector"(5) -> ()
            n158 = Number To Decimal String(number=w337) -> (decimal integer string=w338:string)  [unwired: 1 in]
            n159 = call-poly "Send Message.vi"("error in (no error)"=w341, "event buffer"=w338, "event"="multipleGraphs") -> ("error out"=w340:errorcluster)  [unwired: 8 in]
          }
          event "Tab Control": Value Change {
            n160 = event-data() -> ("NewVal"=w349:enum32{"TCs", "Graphs", "Thermal Profile"})  [unwired: 1 in, 5 out]
            n161 = Equal?(x=w349, y=enum16{"Graphs"}."Graphs") -> (x = y?=w347:bool)
            n162 = case shown="True" w347 {
              tunnel: w346 -> [w351 w353]
              tunnel: [w351 w352] -> w345
              frame False {
              }
              frame True {
                n163 = call-poly "Send Message.vi"("error in (no error)"=w353, "event"="getGraphs") -> ("error out"=w352:errorcluster)  [unwired: 9 in]
              }
            }
          }
          event "Thermocouples": Mouse Down {
            n164 = event-data() -> ("CtlRef"=w365:refnum<vi>, "Coords"=w370:T13)  [unwired: 1 in, 3 out]
            n165 = Unbundle By Name(w370) -> ("Horizontal"=w368:i32, "Vertical"=w367:i32)
            n166 = Add(x=783 ("y"), y=w360) -> (x+y=w355:i32)
            n167 = Less?(x=w368, y=w355) -> (x < y?=w369:bool)
            n168 = Add(x=w357, y=854) -> (x+y=w356:i32)
            n169 = Less?(x=w367, y=w356) -> (x < y?=w366:bool)
            n170 = And(x=w369, y=w366) -> (x .and. y?=w364:bool)
            n171 = case shown="True" w364 {
              tunnel: w365 -> [_ w412]
              tunnel: w363 -> [_ w384]
              tunnel: w363 -> [w371 w382]
              tunnel: [w371 w374] -> w362
              tunnel: w360 -> [_ w373]
              tunnel: w357 -> [_ w372]
              frame False {
              }
              frame True {
                w406 = u16 0 items=["User Selection", "Graph All Thermocouples", "Clear Graph"] ("Graphing Selection")
                n172 = property class="Arr (strict)"(reference=w412) -> ("Array Element.Position"=w404:T12)  [unwired: 1 in, 2 out]
                n173 = local write "Graphing Selection"(w406) -> ()
                n174 = Unbundle By Name(w404) -> ("Left"=w402:i32, "Top"=w405:i32)
                n175 = property on="Thermocouples" class="Arr (strict)"() -> ("Index Values"=w396:u32[])  [unwired: 2 in, 2 out]
                n176 = Subtract(x=w373, y=w402) -> (x-y=w401:i32)
                n177 = Subtract(x=w372, y=w405) -> (x-y=w393:i32)
                n178 = Absolute Value(x=w393) -> (abs(x)=w403:i32)
                n179 = Index Array(array=w396, index=0) -> (element=w392:u32)
                n180 = To Byte Integer(number=w392) -> (8bit integer=w391:i8)
                n181 = Absolute Value(x=w401) -> (abs(x)=w400:i32)
                n182 = local read "Thermocouples"() -> (w375:T3)
                n183 = Quotient & Remainder(x=w403, y=42) -> (floor(x/y)=w390:i32)  [unwired: 1 out]
                n184 = Add(x=w391, y=w390) -> (x+y=w377:i32)
                n185 = Quotient & Remainder(x=w400, y=197 ("Numeric 2")) -> (floor(x/y)=w376:i32)  [unwired: 1 out]
                n186 = Index Array(array=w375, index (row)=w377, index (col)=w376) -> (element=w378:T7)
                n187 = Multiply(x=4, y=w377) -> (x*y=w397:i32)
                n188 = Unbundle By Name(w384) -> ("working array"=w383:bool[])  [unwired: 1 out]
                n189 = Unbundle By Name(w378) -> ("Alarm Color"=w410:u32, "Graph On/Off"=w409:u32, "TC Label"=w408:string, "PlotColor"=w389:u32, "Alarm Status"=w407:string, "Temperature"=w380:string)
                n190 = Add(x=w397, y=w376) -> (x+y=w386:i32)
                n191 = control-ref of="Waveform Chart"() -> (w411:refnum<vi>)
                n192 = Index Array(array=w383, index=w386) -> (element=w385:bool)
                n193 = Decimal String To Number(string=w380) -> ()  [unwired: 2 in, 2 out]
                n194 = Equal?(x=w409, y=u32 12369084) -> (x = y?=w387:bool)
                n195 = case shown="True" w385 {
                  selector: w385 -> [_ w418]
                  tunnel: w411 -> [_ w424]
                  tunnel: w410 -> [_ w423]
                  tunnel: w408 -> [_ w422]
                  tunnel: w407 -> [_ w421]
                  tunnel: w386 -> [_ w414]
                  tunnel: w389 -> [_ w420]
                  tunnel: w387 -> [_ w419]
                  tunnel: w380 -> [_ w417]
                  tunnel: [w413 w416] -> w379
                  tunnel: w378 -> [w413 w415]
                  frame False {
                  }
                  frame True {
                    n196 = case shown="True" w419 {
                      tunnel: w424 -> [w434 w445]
                      tunnel: w423 -> [w428 w440]
                      tunnel: w422 -> [w429 w439]
                      tunnel: w421 -> [w430 w441]
                      tunnel: w420 -> [_ w443]
                      tunnel: w418 -> [_ _]
                      tunnel: w417 -> [w431 w442]
                      tunnel: [w426 w438] -> w416
                      tunnel: w415 -> [w427 w437]
                      tunnel: w414 -> [w425 w436]
                      frame False {
                        w432 = u32 12369084
                        n197 = property on="Property Node" class="WFChart (strict)"(reference=w434, "Active Plot"=w425) -> (reference out=w435:refnum<vi>)  [unwired: 1 in, 1 out]
                        n198 = Bundle By Name(cluster=w427, "Graph On/Off"=w432, "TC Label"=w429, "PlotColor"=w432, "Temperature"=w431, "Alarm Color"=w428, "Alarm Status"=w430) -> (w426:T7)
                        n199 = property class="WFChart (strict)"(reference=w435, "Plot.Visible?"=FALSE ("Plot.Visible")) -> ()  [unwired: 1 in, 2 out]
                      }
                      frame True {
                        n200 = property class="WFChart (strict)"(reference=w445, "Active Plot"=w436) -> (reference out=w446:refnum<vi>)  [unwired: 1 in, 1 out]
                        n201 = Bundle By Name(cluster=w437, "Graph On/Off"=u32 6618880, "TC Label"=w439, "PlotColor"=w443, "Temperature"=w442, "Alarm Color"=w440, "Alarm Status"=w441) -> (w438:T7)
                        n202 = property class="WFChart (strict)"(reference=w446, "Plot.Visible?"=TRUE ("Plot.Visible")) -> ()  [unwired: 1 in, 2 out]
                      }
                    }
                  }
                }
                n203 = Replace Array Subset(array=w375, new element=w379, index (row)=w377, index (col)=w376) -> (w381:T3)
                n204 = Bundle By Name(cluster=w382, "Thermocouples"=w381) -> (w374:T6)
              }
            }
          }
          event "Graphing Selection": Value Change {
            n205 = event-data() -> ("NewVal"=w455:u16)  [unwired: 1 in, 5 out]
            n206 = Unbundle By Name(w450) -> ("Thermocouples"=w449:T3, "working array"=w452:bool[])
            n207 = control-ref of="Waveform Chart"() -> (w456:refnum<vi>)
            n208 = case shown="1" w455 {
              tunnel: w449 -> [w457 w462 w493]
              tunnel: w456 -> [_ w461 w492]
              tunnel: 120 ("disabled index (col)") -> [_ w460 w491]
              tunnel: w450 -> [_ _ _]
              tunnel: w452 -> [_ w459 _]
              tunnel: [w457 w458 w490] -> w451
              frame 0, Default {
              }
              frame 1 {
                n209 = for {
                  N: w460 -> [_]
                  tunnel: w461 -> [w468]
                  shift-right: [w463] -> w458
                  shift-left: w462 -> [w467]
                  tunnel: w459 -> [w464]
                  i -> [w466]
                  n210 = Index Array(array=w464, index=w466) -> (element=w465:bool)
                  n211 = case shown="True" w465 {
                    tunnel: w468 -> [_ w489]
                    tunnel: w467 -> [w469 w470]
                    tunnel: [w469 w471] -> w463
                    tunnel: w466 -> [_ w488]
                    frame False {
                    }
                    frame True {
                      n212 = Quotient & Remainder(x=w488, y=4) -> (x-y*floor(x/y)=w474:i32, floor(x/y)=w473:i32)
                      n213 = Multiply(x=4, y=w473) -> (x*y=w484:i32)
                      n214 = Add(x=w484, y=w474) -> (x+y=w483:i32)
                      n215 = property class="WFChart (strict)"(reference=w489, "Active Plot"=w483) -> (reference out=w486:refnum<vi>)  [unwired: 1 in, 1 out]
                      n216 = Index Array(array=w470, index (row)=w473, index (col)=w474) -> (element=w472:T7)
                      n217 = Unbundle By Name(w472) -> ("TC Label"=w475:string, "Alarm Status"=w481:string, "Temperature"=w480:string, "PlotColor"=w477:u32, "Alarm Color"=w476:u32)
                      n218 = property class="WFChart (strict)"(reference=w486, "Plot.Visible?"=TRUE ("Plot.Visible")) -> ()  [unwired: 1 in, 2 out]
                      n219 = Bundle By Name(cluster=w472, "TC Label"=w475, "Alarm Status"=w481, "Alarm Color"=w476, "Temperature"=w480, "PlotColor"=w477, "Graph On/Off"=u32 6618880) -> (w479:T7)
                      n220 = Replace Array Subset(array=w470, new element=w479, index (row)=w473, index (col)=w474) -> (w471:T3)
                    }
                  }
                }
              }
              frame 2 {
                n221 = for {
                  N: w491 -> [_]
                  tunnel: w492 -> [w511]
                  shift-right: [w494] -> w490
                  shift-left: w493 -> [w498]
                  i -> [w512]
                  w504 = u32 12369084
                  n222 = local read "working array"() -> (w513:bool[])
                  n223 = Quotient & Remainder(x=w512, y=4 ("Numeric")) -> (x-y*floor(x/y)=w496:i32, floor(x/y)=w495:i32)
                  n224 = Index Array(array=w498, index (row)=w495, index (col)=w496) -> (element=w503:T7)
                  n225 = Multiply(x=4, y=w495) -> (x*y=w507:i32)
                  n226 = Add(x=w507, y=w496) -> (x+y=w506:i32)
                  n227 = Index Array(array=w513, index=w512) -> ()  [unwired: 1 out]
                  n228 = property class="WFChart (strict)"(reference=w511, "Active Plot"=w506) -> (reference out=w509:refnum<vi>)  [unwired: 1 in, 1 out]
                  n229 = Unbundle By Name(w503) -> ("TC Label"=w502:string, "Alarm Status"=w501:string, "Temperature"=w500:string, "PlotColor"=w499:u32)
                  n230 = property class="WFChart (strict)"(reference=w509, "Plot.Visible?"=FALSE ("Plot.Visible")) -> ()  [unwired: 1 in, 2 out]
                  n231 = Bundle By Name(cluster=w503, "TC Label"=w502, "Alarm Status"=w501, "Alarm Color"=w504, "Temperature"=w500, "PlotColor"=w499, "Graph On/Off"=w504) -> (w497:T7)
                  n232 = Replace Array Subset(array=w498, new element=w497, index (row)=w495, index (col)=w496) -> (w494:T3)
                }
              }
            }
            n233 = Bundle By Name(cluster=w450, "Thermocouples"=w451) -> (w448:T6)
          }
          event "Set Time TC Graph": Mouse Down {
            n234 = event-data() -> ()  [unwired: 1 in, 8 out]
            n235 = local read "Log/Linear Y-Axis"() -> (w515:u16)
            n236 = control-ref of="Waveform Chart"() -> (w514:refnum<vi>)
            n237 = property on="Property Node" class="WFChart (strict)"(reference=w514, "YScale.Mapping Mode"=w515) -> ()  [unwired: 1 in, 2 out]
            n238 = local read "Total Time"() -> (w516:dbl)
            n239 = local read "Time Scale"() -> (w517:u16)
            n240 = case shown="2" w517 {
              tunnel: w514 -> [w522 w541 w560]
              tunnel: w516 -> [w520 w539 w558]
              frame 0, Default {
                n241 = Not Equal To 0?(x=w520) -> (x != 0?=w521:bool)
                n242 = case shown="True" w521 {
                  tunnel: w522 -> [w524 w536]
                  tunnel: w520 -> [_ w530]
                  frame False {
                    n243 = property on="Property Node" class="WFChart (strict)"(reference=w524) -> (reference out=w523:refnum<vi>, "XScale.Range"=w529:T14)  [unwired: 1 in, 1 out]
                    n244 = Bundle By Name(cluster=w529, "Minimum"=0.0, "Maximum"=3600.0, "Increment"=60.0) -> (w528:T14)
                    n245 = property on="Property Node" class="WFChart (strict)"(reference=w523, "XScale.Range"=w528) -> ()  [unwired: 1 in, 2 out]
                  }
                  frame True {
                    n246 = property on="Property Node" class="WFChart (strict)"(reference=w536) -> (reference out=w533:refnum<vi>, "XScale.Range"=w538:T14)  [unwired: 1 in, 1 out]
                    n247 = Multiply(x=w530, y=60.0) -> (x*y=w532:dbl)
                    n248 = Bundle By Name(cluster=w538, "Minimum"=0.0, "Maximum"=w532, "Increment"=1.0) -> (w537:T14)
                    n249 = property on="Property Node" class="WFChart (strict)"(reference=w533, "XScale.Range"=w537) -> ()  [unwired: 1 in, 2 out]
                  }
                }
              }
              frame 1 {
                n250 = Not Equal To 0?(x=w539) -> (x != 0?=w540:bool)
                n251 = case shown="True" w540 {
                  tunnel: w541 -> [w543 w553]
                  tunnel: w539 -> [_ w550]
                  frame False {
                    n252 = property on="Property Node" class="WFChart (strict)"(reference=w543) -> (reference out=w542:refnum<vi>, "XScale.Range"=w548:T14)  [unwired: 1 in, 1 out]
                    n253 = Bundle By Name(cluster=w548, "Minimum"=0.0, "Maximum"=43200.0, "Increment"=3600.0) -> (w544:T14)
                    n254 = property on="Property Node" class="WFChart (strict)"(reference=w542, "XScale.Range"=w544) -> ()  [unwired: 1 in, 2 out]
                  }
                  frame True {
                    n255 = Multiply(x=w550, y=3600.0) -> (x*y=w549:dbl)
                    n256 = property on="Property Node" class="WFChart (strict)"(reference=w553) -> (reference out=w552:refnum<vi>, "XScale.Range"=w557:T14)  [unwired: 1 in, 1 out]
                    n257 = Bundle By Name(cluster=w557, "Minimum"=0.0, "Maximum"=w549, "Increment"=3600.0) -> (w554:T14)
                    n258 = property on="Property Node" class="WFChart (strict)"(reference=w552, "XScale.Range"=w554) -> ()  [unwired: 1 in, 2 out]
                  }
                }
              }
              frame 2 {
                n259 = Not Equal To 0?(x=w558) -> (x != 0?=w559:bool)
                n260 = case shown="True" w559 {
                  tunnel: w560 -> [w562 w570]
                  tunnel: w558 -> [_ w568]
                  frame False {
                    n261 = property on="Property Node" class="WFChart (strict)"(reference=w562) -> (reference out=w561:refnum<vi>, "XScale.Range"=w567:T14)  [unwired: 1 in, 1 out]
                    n262 = Bundle By Name(cluster=w567, "Minimum"=0.0, "Maximum"=60.0, "Increment"=1.0) -> (w563:T14)
                    n263 = property on="Property Node" class="WFChart (strict)"(reference=w561, "XScale.Range"=w563) -> ()  [unwired: 1 in, 2 out]
                  }
                  frame True {
                    n264 = property on="Property Node" class="WFChart (strict)"(reference=w570) -> (reference out=w569:refnum<vi>, "XScale.Range"=w574:T14)  [unwired: 1 in, 1 out]
                    n265 = Bundle By Name(cluster=w574, "Minimum"=0.0, "Maximum"=w568, "Increment"=1.0) -> (w571:T14)
                    n266 = property on="Property Node" class="WFChart (strict)"(reference=w569, "XScale.Range"=w571) -> ()  [unwired: 1 in, 2 out]
                  }
                }
              }
            }
          }
          event "Set Time TC Graph 1": Mouse Down {
            n267 = event-data() -> ()  [unwired: 1 in, 8 out]
            n268 = local read "Log/Linear Y-Axis 1"() -> (w576:u16)
            n269 = control-ref of="Custom Chart 1"() -> (w575:refnum<vi>)
            n270 = property on="Property Node" class="WFChart (strict)"(reference=w575, "YScale.Mapping Mode"=w576) -> ()  [unwired: 1 in, 2 out]
            n271 = local read "Total Time 1"() -> (w577:dbl)
            n272 = local read "Time Scale 1"() -> (w578:u16)
            n273 = case shown="2" w578 {
              tunnel: w575 -> [w583 w602 w621]
              tunnel: w577 -> [w581 w600 w619]
              frame 0, Default {
                n274 = Not Equal To 0?(x=w581) -> (x != 0?=w582:bool)
                n275 = case shown="True" w582 {
                  tunnel: w583 -> [w585 w597]
                  tunnel: w581 -> [_ w591]
                  frame False {
                    n276 = property on="Property Node" class="WFChart (strict)"(reference=w585) -> (reference out=w584:refnum<vi>, "XScale.Range"=w590:T14)  [unwired: 1 in, 1 out]
                    n277 = Bundle By Name(cluster=w590, "Minimum"=0.0, "Maximum"=3600.0, "Increment"=60.0) -> (w589:T14)
                    n278 = property on="Property Node" class="WFChart (strict)"(reference=w584, "XScale.Range"=w589) -> ()  [unwired: 1 in, 2 out]
                  }
                  frame True {
                    n279 = property on="Property Node" class="WFChart (strict)"(reference=w597) -> (reference out=w594:refnum<vi>, "XScale.Range"=w599:T14)  [unwired: 1 in, 1 out]
                    n280 = Multiply(x=w591, y=60.0) -> (x*y=w593:dbl)
                    n281 = Bundle By Name(cluster=w599, "Minimum"=0.0, "Maximum"=w593, "Increment"=1.0) -> (w598:T14)
                    n282 = property on="Property Node" class="WFChart (strict)"(reference=w594, "XScale.Range"=w598) -> ()  [unwired: 1 in, 2 out]
                  }
                }
              }
              frame 1 {
                n283 = Not Equal To 0?(x=w600) -> (x != 0?=w601:bool)
                n284 = case shown="True" w601 {
                  tunnel: w602 -> [w604 w614]
                  tunnel: w600 -> [_ w611]
                  frame False {
                    n285 = property on="Property Node" class="WFChart (strict)"(reference=w604) -> (reference out=w603:refnum<vi>, "XScale.Range"=w609:T14)  [unwired: 1 in, 1 out]
                    n286 = Bundle By Name(cluster=w609, "Minimum"=0.0, "Maximum"=43200.0, "Increment"=3600.0) -> (w605:T14)
                    n287 = property on="Property Node" class="WFChart (strict)"(reference=w603, "XScale.Range"=w605) -> ()  [unwired: 1 in, 2 out]
                  }
                  frame True {
                    n288 = Multiply(x=w611, y=3600.0) -> (x*y=w610:dbl)
                    n289 = property on="Property Node" class="WFChart (strict)"(reference=w614) -> (reference out=w613:refnum<vi>, "XScale.Range"=w618:T14)  [unwired: 1 in, 1 out]
                    n290 = Bundle By Name(cluster=w618, "Minimum"=0.0, "Maximum"=w610, "Increment"=3600.0) -> (w615:T14)
                    n291 = property on="Property Node" class="WFChart (strict)"(reference=w613, "XScale.Range"=w615) -> ()  [unwired: 1 in, 2 out]
                  }
                }
              }
              frame 2 {
                n292 = Not Equal To 0?(x=w619) -> (x != 0?=w620:bool)
                n293 = case shown="True" w620 {
                  tunnel: w621 -> [w623 w631]
                  tunnel: w619 -> [_ w629]
                  frame False {
                    n294 = property on="Property Node" class="WFChart (strict)"(reference=w623) -> (reference out=w622:refnum<vi>, "XScale.Range"=w628:T14)  [unwired: 1 in, 1 out]
                    n295 = Bundle By Name(cluster=w628, "Minimum"=0.0, "Maximum"=60.0, "Increment"=1.0) -> (w624:T14)
                    n296 = property on="Property Node" class="WFChart (strict)"(reference=w622, "XScale.Range"=w624) -> ()  [unwired: 1 in, 2 out]
                  }
                  frame True {
                    n297 = property on="Property Node" class="WFChart (strict)"(reference=w631) -> (reference out=w630:refnum<vi>, "XScale.Range"=w635:T14)  [unwired: 1 in, 1 out]
                    n298 = Bundle By Name(cluster=w635, "Minimum"=0.0, "Maximum"=w629, "Increment"=1.0) -> (w632:T14)
                    n299 = property on="Property Node" class="WFChart (strict)"(reference=w630, "XScale.Range"=w632) -> ()  [unwired: 1 in, 2 out]
                  }
                }
              }
            }
          }
          event "Set Time TC Graph 2": Mouse Down {
            n300 = event-data() -> ()  [unwired: 1 in, 8 out]
            n301 = local read "Log/Linear Y-Axis 2"() -> (w637:u16)
            n302 = control-ref of="Custom Chart 2"() -> (w636:refnum<vi>)
            n303 = property on="Property Node" class="WFChart (strict)"(reference=w636, "YScale.Mapping Mode"=w637) -> ()  [unwired: 1 in, 2 out]
            n304 = local read "Total Time 2"() -> (w638:dbl)
            n305 = local read "Time Scale 2"() -> (w639:u16)
            n306 = case shown="2" w639 {
              tunnel: w636 -> [w644 w663 w682]
              tunnel: w638 -> [w642 w661 w680]
              frame 0, Default {
                n307 = Not Equal To 0?(x=w642) -> (x != 0?=w643:bool)
                n308 = case shown="True" w643 {
                  tunnel: w644 -> [w646 w658]
                  tunnel: w642 -> [_ w652]
                  frame False {
                    n309 = property on="Property Node" class="WFChart (strict)"(reference=w646) -> (reference out=w645:refnum<vi>, "XScale.Range"=w651:T14)  [unwired: 1 in, 1 out]
                    n310 = Bundle By Name(cluster=w651, "Minimum"=0.0, "Maximum"=3600.0, "Increment"=60.0) -> (w650:T14)
                    n311 = property on="Property Node" class="WFChart (strict)"(reference=w645, "XScale.Range"=w650) -> ()  [unwired: 1 in, 2 out]
                  }
                  frame True {
                    n312 = property on="Property Node" class="WFChart (strict)"(reference=w658) -> (reference out=w655:refnum<vi>, "XScale.Range"=w660:T14)  [unwired: 1 in, 1 out]
                    n313 = Multiply(x=w652, y=60.0) -> (x*y=w654:dbl)
                    n314 = Bundle By Name(cluster=w660, "Minimum"=0.0, "Maximum"=w654, "Increment"=1.0) -> (w659:T14)
                    n315 = property on="Property Node" class="WFChart (strict)"(reference=w655, "XScale.Range"=w659) -> ()  [unwired: 1 in, 2 out]
                  }
                }
              }
              frame 1 {
                n316 = Not Equal To 0?(x=w661) -> (x != 0?=w662:bool)
                n317 = case shown="True" w662 {
                  tunnel: w663 -> [w665 w675]
                  tunnel: w661 -> [_ w672]
                  frame False {
                    n318 = property on="Property Node" class="WFChart (strict)"(reference=w665) -> (reference out=w664:refnum<vi>, "XScale.Range"=w670:T14)  [unwired: 1 in, 1 out]
                    n319 = Bundle By Name(cluster=w670, "Minimum"=0.0, "Maximum"=43200.0, "Increment"=3600.0) -> (w666:T14)
                    n320 = property on="Property Node" class="WFChart (strict)"(reference=w664, "XScale.Range"=w666) -> ()  [unwired: 1 in, 2 out]
                  }
                  frame True {
                    n321 = Multiply(x=w672, y=3600.0) -> (x*y=w671:dbl)
                    n322 = property on="Property Node" class="WFChart (strict)"(reference=w675) -> (reference out=w674:refnum<vi>, "XScale.Range"=w679:T14)  [unwired: 1 in, 1 out]
                    n323 = Bundle By Name(cluster=w679, "Minimum"=0.0, "Maximum"=w671, "Increment"=3600.0) -> (w676:T14)
                    n324 = property on="Property Node" class="WFChart (strict)"(reference=w674, "XScale.Range"=w676) -> ()  [unwired: 1 in, 2 out]
                  }
                }
              }
              frame 2 {
                n325 = Not Equal To 0?(x=w680) -> (x != 0?=w681:bool)
                n326 = case shown="True" w681 {
                  tunnel: w682 -> [w684 w692]
                  tunnel: w680 -> [_ w690]
                  frame False {
                    n327 = property on="Property Node" class="WFChart (strict)"(reference=w684) -> (reference out=w683:refnum<vi>, "XScale.Range"=w689:T14)  [unwired: 1 in, 1 out]
                    n328 = Bundle By Name(cluster=w689, "Minimum"=0.0, "Maximum"=60.0, "Increment"=1.0) -> (w685:T14)
                    n329 = property on="Property Node" class="WFChart (strict)"(reference=w683, "XScale.Range"=w685) -> ()  [unwired: 1 in, 2 out]
                  }
                  frame True {
                    n330 = property on="Property Node" class="WFChart (strict)"(reference=w692) -> (reference out=w691:refnum<vi>, "XScale.Range"=w696:T14)  [unwired: 1 in, 1 out]
                    n331 = Bundle By Name(cluster=w696, "Minimum"=0.0, "Maximum"=w690, "Increment"=1.0) -> (w693:T14)
                    n332 = property on="Property Node" class="WFChart (strict)"(reference=w691, "XScale.Range"=w693) -> ()  [unwired: 1 in, 2 out]
                  }
                }
              }
            }
          }
          event "Set Time TC Graph 3": Mouse Down {
            n333 = event-data() -> ()  [unwired: 1 in, 8 out]
            n334 = local read "Log/Linear Y-Axis 3"() -> (w698:u16)
            n335 = control-ref of="Custom Chart 3"() -> (w697:refnum<vi>)
            n336 = property on="Property Node" class="WFChart (strict)"(reference=w697, "YScale.Mapping Mode"=w698) -> ()  [unwired: 1 in, 2 out]
            n337 = local read "Total Time 3"() -> (w699:dbl)
            n338 = local read "Time Scale 3"() -> (w700:u16)
            n339 = case shown="2" w700 {
              tunnel: w697 -> [w705 w724 w743]
              tunnel: w699 -> [w703 w722 w741]
              frame 0, Default {
                n340 = Not Equal To 0?(x=w703) -> (x != 0?=w704:bool)
                n341 = case shown="True" w704 {
                  tunnel: w705 -> [w707 w719]
                  tunnel: w703 -> [_ w713]
                  frame False {
                    n342 = property on="Property Node" class="WFChart (strict)"(reference=w707) -> (reference out=w706:refnum<vi>, "XScale.Range"=w712:T14)  [unwired: 1 in, 1 out]
                    n343 = Bundle By Name(cluster=w712, "Minimum"=0.0, "Maximum"=3600.0, "Increment"=60.0) -> (w711:T14)
                    n344 = property on="Property Node" class="WFChart (strict)"(reference=w706, "XScale.Range"=w711) -> ()  [unwired: 1 in, 2 out]
                  }
                  frame True {
                    n345 = property on="Property Node" class="WFChart (strict)"(reference=w719) -> (reference out=w716:refnum<vi>, "XScale.Range"=w721:T14)  [unwired: 1 in, 1 out]
                    n346 = Multiply(x=w713, y=60.0) -> (x*y=w715:dbl)
                    n347 = Bundle By Name(cluster=w721, "Minimum"=0.0, "Maximum"=w715, "Increment"=1.0) -> (w720:T14)
                    n348 = property on="Property Node" class="WFChart (strict)"(reference=w716, "XScale.Range"=w720) -> ()  [unwired: 1 in, 2 out]
                  }
                }
              }
              frame 1 {
                n349 = Not Equal To 0?(x=w722) -> (x != 0?=w723:bool)
                n350 = case shown="True" w723 {
                  tunnel: w724 -> [w726 w736]
                  tunnel: w722 -> [_ w733]
                  frame False {
                    n351 = property on="Property Node" class="WFChart (strict)"(reference=w726) -> (reference out=w725:refnum<vi>, "XScale.Range"=w731:T14)  [unwired: 1 in, 1 out]
                    n352 = Bundle By Name(cluster=w731, "Minimum"=0.0, "Maximum"=43200.0, "Increment"=3600.0) -> (w727:T14)
                    n353 = property on="Property Node" class="WFChart (strict)"(reference=w725, "XScale.Range"=w727) -> ()  [unwired: 1 in, 2 out]
                  }
                  frame True {
                    n354 = Multiply(x=w733, y=3600.0) -> (x*y=w732:dbl)
                    n355 = property on="Property Node" class="WFChart (strict)"(reference=w736) -> (reference out=w735:refnum<vi>, "XScale.Range"=w740:T14)  [unwired: 1 in, 1 out]
                    n356 = Bundle By Name(cluster=w740, "Minimum"=0.0, "Maximum"=w732, "Increment"=3600.0) -> (w737:T14)
                    n357 = property on="Property Node" class="WFChart (strict)"(reference=w735, "XScale.Range"=w737) -> ()  [unwired: 1 in, 2 out]
                  }
                }
              }
              frame 2 {
                n358 = Not Equal To 0?(x=w741) -> (x != 0?=w742:bool)
                n359 = case shown="True" w742 {
                  tunnel: w743 -> [w745 w753]
                  tunnel: w741 -> [_ w751]
                  frame False {
                    n360 = property on="Property Node" class="WFChart (strict)"(reference=w745) -> (reference out=w744:refnum<vi>, "XScale.Range"=w750:T14)  [unwired: 1 in, 1 out]
                    n361 = Bundle By Name(cluster=w750, "Minimum"=0.0, "Maximum"=60.0, "Increment"=1.0) -> (w746:T14)
                    n362 = property on="Property Node" class="WFChart (strict)"(reference=w744, "XScale.Range"=w746) -> ()  [unwired: 1 in, 2 out]
                  }
                  frame True {
                    n363 = property on="Property Node" class="WFChart (strict)"(reference=w753) -> (reference out=w752:refnum<vi>, "XScale.Range"=w757:T14)  [unwired: 1 in, 1 out]
                    n364 = Bundle By Name(cluster=w757, "Minimum"=0.0, "Maximum"=w751, "Increment"=1.0) -> (w754:T14)
                    n365 = property on="Property Node" class="WFChart (strict)"(reference=w752, "XScale.Range"=w754) -> ()  [unwired: 1 in, 2 out]
                  }
                }
              }
            }
          }
          event "Set Time TC Graph 4": Mouse Down {
            n366 = event-data() -> ()  [unwired: 1 in, 8 out]
            n367 = local read "Log/Linear Y-Axis 4"() -> (w759:u16)
            n368 = control-ref of="Custom Chart 4"() -> (w758:refnum<vi>)
            n369 = property on="Property Node" class="WFChart (strict)"(reference=w758, "YScale.Mapping Mode"=w759) -> ()  [unwired: 1 in, 2 out]
            n370 = local read "Total Time 4"() -> (w760:dbl)
            n371 = local read "Time Scale 4"() -> (w761:u16)
            n372 = case shown="2" w761 {
              tunnel: w758 -> [w766 w785 w804]
              tunnel: w760 -> [w764 w783 w802]
              frame 0, Default {
                n373 = Not Equal To 0?(x=w764) -> (x != 0?=w765:bool)
                n374 = case shown="True" w765 {
                  tunnel: w766 -> [w768 w780]
                  tunnel: w764 -> [_ w774]
                  frame False {
                    n375 = property on="Property Node" class="WFChart (strict)"(reference=w768) -> (reference out=w767:refnum<vi>, "XScale.Range"=w773:T14)  [unwired: 1 in, 1 out]
                    n376 = Bundle By Name(cluster=w773, "Minimum"=0.0, "Maximum"=3600.0, "Increment"=60.0) -> (w772:T14)
                    n377 = property on="Property Node" class="WFChart (strict)"(reference=w767, "XScale.Range"=w772) -> ()  [unwired: 1 in, 2 out]
                  }
                  frame True {
                    n378 = property on="Property Node" class="WFChart (strict)"(reference=w780) -> (reference out=w777:refnum<vi>, "XScale.Range"=w782:T14)  [unwired: 1 in, 1 out]
                    n379 = Multiply(x=w774, y=60.0) -> (x*y=w776:dbl)
                    n380 = Bundle By Name(cluster=w782, "Minimum"=0.0, "Maximum"=w776, "Increment"=1.0) -> (w781:T14)
                    n381 = property on="Property Node" class="WFChart (strict)"(reference=w777, "XScale.Range"=w781) -> ()  [unwired: 1 in, 2 out]
                  }
                }
              }
              frame 1 {
                n382 = Not Equal To 0?(x=w783) -> (x != 0?=w784:bool)
                n383 = case shown="True" w784 {
                  tunnel: w785 -> [w787 w797]
                  tunnel: w783 -> [_ w794]
                  frame False {
                    n384 = property on="Property Node" class="WFChart (strict)"(reference=w787) -> (reference out=w786:refnum<vi>, "XScale.Range"=w792:T14)  [unwired: 1 in, 1 out]
                    n385 = Bundle By Name(cluster=w792, "Minimum"=0.0, "Maximum"=43200.0, "Increment"=3600.0) -> (w788:T14)
                    n386 = property on="Property Node" class="WFChart (strict)"(reference=w786, "XScale.Range"=w788) -> ()  [unwired: 1 in, 2 out]
                  }
                  frame True {
                    n387 = Multiply(x=w794, y=3600.0) -> (x*y=w793:dbl)
                    n388 = property on="Property Node" class="WFChart (strict)"(reference=w797) -> (reference out=w796:refnum<vi>, "XScale.Range"=w801:T14)  [unwired: 1 in, 1 out]
                    n389 = Bundle By Name(cluster=w801, "Minimum"=0.0, "Maximum"=w793, "Increment"=3600.0) -> (w798:T14)
                    n390 = property on="Property Node" class="WFChart (strict)"(reference=w796, "XScale.Range"=w798) -> ()  [unwired: 1 in, 2 out]
                  }
                }
              }
              frame 2 {
                n391 = Not Equal To 0?(x=w802) -> (x != 0?=w803:bool)
                n392 = case shown="True" w803 {
                  tunnel: w804 -> [w806 w814]
                  tunnel: w802 -> [_ w812]
                  frame False {
                    n393 = property on="Property Node" class="WFChart (strict)"(reference=w806) -> (reference out=w805:refnum<vi>, "XScale.Range"=w811:T14)  [unwired: 1 in, 1 out]
                    n394 = Bundle By Name(cluster=w811, "Minimum"=0.0, "Maximum"=60.0, "Increment"=1.0) -> (w807:T14)
                    n395 = property on="Property Node" class="WFChart (strict)"(reference=w805, "XScale.Range"=w807) -> ()  [unwired: 1 in, 2 out]
                  }
                  frame True {
                    n396 = property on="Property Node" class="WFChart (strict)"(reference=w814) -> (reference out=w813:refnum<vi>, "XScale.Range"=w818:T14)  [unwired: 1 in, 1 out]
                    n397 = Bundle By Name(cluster=w818, "Minimum"=0.0, "Maximum"=w812, "Increment"=1.0) -> (w815:T14)
                    n398 = property on="Property Node" class="WFChart (strict)"(reference=w813, "XScale.Range"=w815) -> ()  [unwired: 1 in, 2 out]
                  }
                }
              }
            }
          }
          event "Set Time TC Graph 5": Mouse Down {
            n399 = event-data() -> ()  [unwired: 1 in, 8 out]
            n400 = local read "Log/Linear Y-Axis 5"() -> (w820:u16)
            n401 = control-ref of="Custom Chart 5"() -> (w819:refnum<vi>)
            n402 = property on="Property Node" class="WFChart (strict)"(reference=w819, "YScale.Mapping Mode"=w820) -> ()  [unwired: 1 in, 2 out]
            n403 = local read "Total Time 5"() -> (w821:dbl)
            n404 = local read "Time Scale 5"() -> (w822:u16)
            n405 = case shown="2" w822 {
              tunnel: w819 -> [w827 w846 w865]
              tunnel: w821 -> [w825 w844 w863]
              frame 0, Default {
                n406 = Not Equal To 0?(x=w825) -> (x != 0?=w826:bool)
                n407 = case shown="True" w826 {
                  tunnel: w827 -> [w829 w841]
                  tunnel: w825 -> [_ w835]
                  frame False {
                    n408 = property on="Property Node" class="WFChart (strict)"(reference=w829) -> (reference out=w828:refnum<vi>, "XScale.Range"=w834:T14)  [unwired: 1 in, 1 out]
                    n409 = Bundle By Name(cluster=w834, "Minimum"=0.0, "Maximum"=3600.0, "Increment"=60.0) -> (w833:T14)
                    n410 = property on="Property Node" class="WFChart (strict)"(reference=w828, "XScale.Range"=w833) -> ()  [unwired: 1 in, 2 out]
                  }
                  frame True {
                    n411 = property on="Property Node" class="WFChart (strict)"(reference=w841) -> (reference out=w838:refnum<vi>, "XScale.Range"=w843:T14)  [unwired: 1 in, 1 out]
                    n412 = Multiply(x=w835, y=60.0) -> (x*y=w837:dbl)
                    n413 = Bundle By Name(cluster=w843, "Minimum"=0.0, "Maximum"=w837, "Increment"=1.0) -> (w842:T14)
                    n414 = property on="Property Node" class="WFChart (strict)"(reference=w838, "XScale.Range"=w842) -> ()  [unwired: 1 in, 2 out]
                  }
                }
              }
              frame 1 {
                n415 = Not Equal To 0?(x=w844) -> (x != 0?=w845:bool)
                n416 = case shown="True" w845 {
                  tunnel: w846 -> [w848 w858]
                  tunnel: w844 -> [_ w855]
                  frame False {
                    n417 = property on="Property Node" class="WFChart (strict)"(reference=w848) -> (reference out=w847:refnum<vi>, "XScale.Range"=w853:T14)  [unwired: 1 in, 1 out]
                    n418 = Bundle By Name(cluster=w853, "Minimum"=0.0, "Maximum"=43200.0, "Increment"=3600.0) -> (w849:T14)
                    n419 = property on="Property Node" class="WFChart (strict)"(reference=w847, "XScale.Range"=w849) -> ()  [unwired: 1 in, 2 out]
                  }
                  frame True {
                    n420 = Multiply(x=w855, y=3600.0) -> (x*y=w854:dbl)
                    n421 = property on="Property Node" class="WFChart (strict)"(reference=w858) -> (reference out=w857:refnum<vi>, "XScale.Range"=w862:T14)  [unwired: 1 in, 1 out]
                    n422 = Bundle By Name(cluster=w862, "Minimum"=0.0, "Maximum"=w854, "Increment"=3600.0) -> (w859:T14)
                    n423 = property on="Property Node" class="WFChart (strict)"(reference=w857, "XScale.Range"=w859) -> ()  [unwired: 1 in, 2 out]
                  }
                }
              }
              frame 2 {
                n424 = Not Equal To 0?(x=w863) -> (x != 0?=w864:bool)
                n425 = case shown="True" w864 {
                  tunnel: w865 -> [w867 w875]
                  tunnel: w863 -> [_ w873]
                  frame False {
                    n426 = property on="Property Node" class="WFChart (strict)"(reference=w867) -> (reference out=w866:refnum<vi>, "XScale.Range"=w872:T14)  [unwired: 1 in, 1 out]
                    n427 = Bundle By Name(cluster=w872, "Minimum"=0.0, "Maximum"=60.0, "Increment"=1.0) -> (w868:T14)
                    n428 = property on="Property Node" class="WFChart (strict)"(reference=w866, "XScale.Range"=w868) -> ()  [unwired: 1 in, 2 out]
                  }
                  frame True {
                    n429 = property on="Property Node" class="WFChart (strict)"(reference=w875) -> (reference out=w874:refnum<vi>, "XScale.Range"=w879:T14)  [unwired: 1 in, 1 out]
                    n430 = Bundle By Name(cluster=w879, "Minimum"=0.0, "Maximum"=w873, "Increment"=1.0) -> (w876:T14)
                    n431 = property on="Property Node" class="WFChart (strict)"(reference=w874, "XScale.Range"=w876) -> ()  [unwired: 1 in, 2 out]
                  }
                }
              }
            }
          }
          event "Set Time TC Graph 6": Mouse Down {
            n432 = event-data() -> ()  [unwired: 1 in, 8 out]
            n433 = local read "Log/Linear Y-Axis 6"() -> (w881:u16)
            n434 = control-ref of="Custom Chart 6"() -> (w880:refnum<vi>)
            n435 = property on="Property Node" class="WFChart (strict)"(reference=w880, "YScale.Mapping Mode"=w881) -> ()  [unwired: 1 in, 2 out]
            n436 = local read "Total Time 6"() -> (w882:dbl)
            n437 = local read "Time Scale 6"() -> (w883:u16)
            n438 = case shown="2" w883 {
              tunnel: w880 -> [w888 w907 w926]
              tunnel: w882 -> [w886 w905 w924]
              frame 0, Default {
                n439 = Not Equal To 0?(x=w886) -> (x != 0?=w887:bool)
                n440 = case shown="True" w887 {
                  tunnel: w888 -> [w890 w902]
                  tunnel: w886 -> [_ w896]
                  frame False {
                    n441 = property on="Property Node" class="WFChart (strict)"(reference=w890) -> (reference out=w889:refnum<vi>, "XScale.Range"=w895:T14)  [unwired: 1 in, 1 out]
                    n442 = Bundle By Name(cluster=w895, "Minimum"=0.0, "Maximum"=3600.0, "Increment"=60.0) -> (w894:T14)
                    n443 = property on="Property Node" class="WFChart (strict)"(reference=w889, "XScale.Range"=w894) -> ()  [unwired: 1 in, 2 out]
                  }
                  frame True {
                    n444 = property on="Property Node" class="WFChart (strict)"(reference=w902) -> (reference out=w899:refnum<vi>, "XScale.Range"=w904:T14)  [unwired: 1 in, 1 out]
                    n445 = Multiply(x=w896, y=60.0) -> (x*y=w898:dbl)
                    n446 = Bundle By Name(cluster=w904, "Minimum"=0.0, "Maximum"=w898, "Increment"=1.0) -> (w903:T14)
                    n447 = property on="Property Node" class="WFChart (strict)"(reference=w899, "XScale.Range"=w903) -> ()  [unwired: 1 in, 2 out]
                  }
                }
              }
              frame 1 {
                n448 = Not Equal To 0?(x=w905) -> (x != 0?=w906:bool)
                n449 = case shown="True" w906 {
                  tunnel: w907 -> [w909 w919]
                  tunnel: w905 -> [_ w916]
                  frame False {
                    n450 = property on="Property Node" class="WFChart (strict)"(reference=w909) -> (reference out=w908:refnum<vi>, "XScale.Range"=w914:T14)  [unwired: 1 in, 1 out]
                    n451 = Bundle By Name(cluster=w914, "Minimum"=0.0, "Maximum"=43200.0, "Increment"=3600.0) -> (w910:T14)
                    n452 = property on="Property Node" class="WFChart (strict)"(reference=w908, "XScale.Range"=w910) -> ()  [unwired: 1 in, 2 out]
                  }
                  frame True {
                    n453 = Multiply(x=w916, y=3600.0) -> (x*y=w915:dbl)
                    n454 = property on="Property Node" class="WFChart (strict)"(reference=w919) -> (reference out=w918:refnum<vi>, "XScale.Range"=w923:T14)  [unwired: 1 in, 1 out]
                    n455 = Bundle By Name(cluster=w923, "Minimum"=0.0, "Maximum"=w915, "Increment"=3600.0) -> (w920:T14)
                    n456 = property on="Property Node" class="WFChart (strict)"(reference=w918, "XScale.Range"=w920) -> ()  [unwired: 1 in, 2 out]
                  }
                }
              }
              frame 2 {
                n457 = Not Equal To 0?(x=w924) -> (x != 0?=w925:bool)
                n458 = case shown="True" w925 {
                  tunnel: w926 -> [w928 w936]
                  tunnel: w924 -> [_ w934]
                  frame False {
                    n459 = property on="Property Node" class="WFChart (strict)"(reference=w928) -> (reference out=w927:refnum<vi>, "XScale.Range"=w933:T14)  [unwired: 1 in, 1 out]
                    n460 = Bundle By Name(cluster=w933, "Minimum"=0.0, "Maximum"=60.0, "Increment"=1.0) -> (w929:T14)
                    n461 = property on="Property Node" class="WFChart (strict)"(reference=w927, "XScale.Range"=w929) -> ()  [unwired: 1 in, 2 out]
                  }
                  frame True {
                    n462 = property on="Property Node" class="WFChart (strict)"(reference=w936) -> (reference out=w935:refnum<vi>, "XScale.Range"=w940:T14)  [unwired: 1 in, 1 out]
                    n463 = Bundle By Name(cluster=w940, "Minimum"=0.0, "Maximum"=w934, "Increment"=1.0) -> (w937:T14)
                    n464 = property on="Property Node" class="WFChart (strict)"(reference=w935, "XScale.Range"=w937) -> ()  [unwired: 1 in, 2 out]
                  }
                }
              }
            }
          }
          event "exit": Value Change {
            n465 = event-data() -> ()  [unwired: 1 in, 1 out]
            n466 = call "Deliver Message.vi"("error in (no error)"=w943, "event"="exit") -> ("error out"=w941:errorcluster)  [unwired: 9 in]
          }
        }
      }
      frame "getPressure" {
        n467 = Unbundle By Name(w950) -> ("Http session"=w959:T5, "URL prefex"=w957:string)
        n468 = Build Array(3, 2, 1) -> (w955:i32[])
        n469 = Flatten To JSON(anything=w955) -> (JSON string=w954:string)  [unwired: 2 in, 1 out]
        n470 = Concatenate Strings(w957, "getPressureGauges" ("url")) -> (w958:string)
        n471 = case shown="True" "Read Pressure Gauges" {
          tunnel: [w962 w970] -> w960
          tunnel: w959 -> [w962 w969]
          tunnel: w958 -> [_ w968]
          tunnel: w954 -> [_ w967]
          tunnel: w949 -> [w961 w965]
          tunnel: [w961 w964] -> w948
          tunnel: [_ w963] -> w946
          frame False {
          }
          frame True {
            n472 = call-poly <vilib>:"POST.vi"("client handle"=w969, "url"=w968, "buffer"=w967, "error in (no error)"=w965) -> ("client handle out"=w970:T5, "body"=w966:string, "error out"=w964:errorcluster)  [unwired: 8 in, 1 out]
            n473 = case shown="Default" w966 {
              selector: w966 -> [_ w976 w979]
              tunnel: [_ w971 _] -> w963
              frame "" {
              }
              frame Default {
                n474 = Unflatten From JSON(JSON string=w976, type and defaults=cluster{"Pressure":dbl[]} {"Pressure"=[]}) -> (value=w978:cluster{"Pressure":dbl[]})  [unwired: 5 in, 1 out]
                n475 = Unbundle By Name(w978) -> ("Pressure"=w971:dbl[])
                n476 = Array To Cluster(array=w971) -> (cluster=w972:T15)
                n477 = Unbundle(w972) -> ("Pressure[0]"=w975:dbl, "Pressure[1]"=w973:dbl, "Pressure[2]"=w974:dbl)
                n478 = Build Array(w975) -> ()  [unwired: 1 out]
                n479 = Build Array(w974) -> ()  [unwired: 1 out]
                n480 = Build Array(w973) -> ()  [unwired: 1 out]
              }
              frame "Buffer Needs to be list" {
                n481 = One Button Dialog(message=w979) -> ()  [unwired: 1 in, 1 out]
              }
            }
          }
        }
        n482 = Bundle By Name(cluster=w950, "Http session"=w960, "Pressure"=w946) -> (w947:T6)
      }
      frame "getTC" {
        w997 = T10 {"time"="", "TCs"=[]} ("Cluster")
        n483 = property on="Waveform Chart" class="WFChart (strict)"("LegScrollVis"=TRUE ("Legend:Scrollbar Visible")) -> ()  [unwired: 2 in, 2 out]
        n484 = local read "Local Debug"() -> (w995:bool)
        n485 = Unbundle By Name(w990) -> ("Http session"=w1004:T5, "URL prefex"=w1002:string)
        n486 = Concatenate Strings(w1002, "getAllThermoCoupleData" ("url")) -> (w1003:string)
        n487 = Flatten To JSON(anything=w997) -> (JSON string=w996:string)  [unwired: 2 in, 1 out]
        n488 = case shown="True" w995 {
          tunnel: w1006 -> [w1081 w1082]
          tunnel: [w1080 w1083] -> w980
          tunnel: [w1079 w1084] -> w1005
          tunnel: w1004 -> [w1078 w1087]
          tunnel: w1003 -> [w1077 w1088]
          tunnel: [w1076 w1085] -> w1000
          tunnel: [w1075 w1086] -> _
          tunnel: w996 -> [_ w1089]
          frame False {
            n489 = call <vilib>:"GET.vi"("client handle"=w1078, "url"=w1077, "error in (no error)"=w1081) -> ("client handle out"=w1079:T5, "headers"=w1075:string, "body"=w1076:string, "error out"=w1080:errorcluster)  [unwired: 9 in]
          }
          frame True {
            n490 = call-poly <vilib>:"POST.vi"("client handle"=w1087, "url"=w1088, "buffer"=w1089, "error in (no error)"=w1082) -> ("client handle out"=w1084:T5, "headers"=w1086:string, "body"=w1085:string, "error out"=w1083:errorcluster)  [unwired: 8 in]
          }
        }
        n491 = Bundle By Name(cluster=w990, "Http session"=w1005) -> (w994:T6)
        n492 = Unflatten From JSON(JSON string=w1000, type and defaults=w997) -> (value=w999:T10)  [unwired: 5 in, 1 out]
        n493 = Unbundle By Name(w999) -> ("TCs"=w986:T11)
        n494 = Unbundle By Name(w994) -> ("working array"=w987:bool[], "Thermocouples"=w988:T3)
        n495 = for {
          N: 120 -> [_]
          tunnel: w986 -> [w1037] mode=indexing
          tunnel: [w1036] -> w981 mode=indexing
          shift-right: [w1015] -> w983
          shift-left: w988 -> [w1022]
          shift-right: [w1014] -> w989
          shift-left: w987 -> [w1013]
          i -> [w1012]
          n496 = Unbundle By Name(w1037) -> ("thermocouple"=w1047:i32, "temp"=w1010:dbl, "alarm"=w1041:i32, "working"=w1040:bool)
          n497 = Quotient & Remainder(x=w1012, y=4) -> (x-y*floor(x/y)=w1020:i32, floor(x/y)=w1021:i32)
          n498 = Index Array(array=w1022, index (row)=w1021, index (col)=w1020) -> (element=w1035:T7)
          n499 = Multiply(x=w1021, y=4) -> (x*y=w1030:i32)
          n500 = Multiply(x=w1021, y=4) -> (x*y=w1042:i32)
          n501 = Unbundle By Name(w1035) -> ("Graph On/Off"=w1019:u32)
          n502 = Add(x=w1030, y=w1020) -> (x+y=w1028:i32)
          n503 = Add(x=w1042, y=w1020) -> (x+y=w1011:i32)
          n504 = Replace Array Subset(array=w1013, new element=w1040, index=w1012) -> (w1014:bool[])
          n505 = To Double Precision Float(number=w1010) -> (double precision float=w1008:dbl)
          n506 = Get Date/Time In Seconds() -> (seconds since 1Jan1904=w1039:timestamp)
          n507 = Random Number (0-1)() -> (number: 0 to 1=w1009:dbl)
          n508 = Add(x=w1009, y=w1008) -> (x+y=w1007:dbl)
          n509 = property on="Waveform Chart" class="WFChart (strict)"("Active Plot"=w1011) -> ()  [unwired: 2 in, 2 out]
          n510 = Index Array(array=w1014, index=w1028) -> (element=w1027:bool)
          n511 = Bundle By Name("t0"=w1039) -> (w1038:waveform(dbl))  [unwired: 1 in]
          n512 = Build Array(w1007) -> (w1045:dbl[])
          n513 = Number To Fractional String(number=w1007, precision (6)=i16 2 ("width (-)")) -> (F-format string=w1025:string)  [unwired: 2 in]
          n514 = Bundle By Name(cluster=w1038, "Y"=w1045) -> (w1036:waveform(dbl))
          n515 = case shown="True" w1027 {
            tunnel: w1019 -> [_ w1052]
            tunnel: [u32 12369084 ("y") w1052] -> w1023
            tunnel: w1025 -> [_ w1051]
            tunnel: ["NaN" w1051] -> w1024
            frame False {
            }
            frame True {
            }
          }
          n516 = case shown="1" w1041 {
            tunnel: ["" "L" "H"] -> w1016
            tunnel: w1041 -> [_ _ _]
            tunnel: [u32 12369084 u32 2812927 u32 16711680] -> w1017
            frame 0, Default {
            }
            frame 1 {
            }
            frame 2 {
            }
          }
          n517 = Number To Decimal String(number=w1047) -> (decimal integer string=w1048:string)  [unwired: 1 in]
          n518 = Index Array(array=w1022, index (row)=w1021, index (col)=w1020) -> (element=w1033:T7)
          n519 = Equal?(x=w1023, y=u32 6618880) -> (x = y?=w1031:bool)
          n520 = Concatenate Strings("TC " ("string"), w1048) -> (w1018:string)
          n521 = property on="Waveform Chart" class="WFChart (strict)"("Plot.Plot Name"=w1018) -> ()  [unwired: 2 in, 2 out]
          n522 = case shown="True" w1031 {
            tunnel: [w1060 w1068] -> w1034
            tunnel: w1033 -> [w1059 w1067]
            tunnel: w1023 -> [w1057 w1066]
            tunnel: w1024 -> [w1058 w1065]
            tunnel: w1018 -> [w1056 w1064]
            tunnel: w1017 -> [w1055 w1063]
            tunnel: w1016 -> [w1054 w1062]
            frame False {
              n523 = Bundle By Name(cluster=w1059, "Graph On/Off"=w1057, "TC Label"=w1056, "PlotColor"=u32 12369084 ("y"), "Temperature"=w1058, "Alarm Color"=w1055, "Alarm Status"=w1054) -> (w1060:T7)
            }
            frame True {
              n524 = property on="Waveform Chart" class="WFChart (strict)"() -> ("Plot.Plot Color"=w1061:u32)  [unwired: 2 in, 2 out]
              n525 = Bundle By Name(cluster=w1067, "Graph On/Off"=w1066, "TC Label"=w1064, "PlotColor"=w1061, "Temperature"=w1065, "Alarm Color"=w1063, "Alarm Status"=w1062) -> (w1068:T7)
            }
          }
          n526 = Replace Array Subset(array=w1022, new element=w1034, index (row)=w1021, index (col)=w1020) -> (w1015:T3)
        }
        n527 = local write "Thermocouples"(w983) -> ()
        n528 = Bundle By Name(cluster=w990, "Thermocouples"=w983, "working array"=w989) -> (w984:T6)
        n529 = Build Array (concatenate)(waveform(dbl) {"t0"=timestamp(0 s since 1904-01-01), "dt"=1.0, "Y"=[]} ("element"), w981) -> (w993:waveform(dbl)[])
        n530 = Delete From Array(array=w993, index=0) -> (array with subset deleted=→"Waveform Chart":waveform(dbl)[])  [unwired: 1 in, 1 out]
      }
      frame "getTemps" {
        n531 = Unbundle By Name(w1094) -> ("Http session"=w1098:T5, "URL prefex"=w1096:string)
        n532 = Concatenate Strings(w1096, "getMCC_json" ("url")) -> (w1097:string)
        n533 = case shown="False" "Read MCC" {
          tunnel: w1098 -> [_ w1106]
          tunnel: w1097 -> [_ w1105]
          tunnel: w1093 -> [_ w1103]
          tunnel: [w1100 w1102] -> w1092
          tunnel: T8 {"Cryopump Stage 1 Temp"=[0.0], "Cryopump Stage 2 Temp"=[0.0], "Compressor Temp"=[0.0]} -> [w1100 w1101]
          frame False {
          }
          frame True {
            n534 = call-poly <vilib>:"POST.vi"("client handle"=w1106, "url"=w1105, "error in (no error)"=w1103) -> ("body"=w1104:string)  [unwired: 9 in, 3 out]
            n535 = case shown="Default" w1104 {
              selector: w1104 -> [_ w1119 w1121]
              tunnel: [_ w1117 _] -> w1102
              tunnel: w1101 -> [_ w1116 _]
              frame "" {
              }
              frame Default {
                n536 = Unflatten From JSON(JSON string=w1119, type and defaults=T9 {"DutyCycle"=0, "Stage1Temp"=0, "CryoPumpReadyState"={"MotorOn"=FALSE, "Ready"=FALSE}, "PurgeValveState"=FALSE, "RegenError"="", "RegenStep"="", "RoughingValveState"=FALSE, "RoughingInterlock"={"RoughingPermission"=FALSE, "RoughingNeeded"=FALSE, "Cryopumprunning"=FALSE}, "Stage2Temp"=0, "Status"={"PumpOn"=FALSE, "RoughOpen"=FALSE, "PurgeOpen"=FALSE, "ThermocoupleGaugeOn"=FALSE, "PowerFailureOccurred"=FALSE}, "TcPressure"=0}) -> (value=w1120:T9)  [unwired: 5 in, 1 out]
                n537 = Unbundle By Name(w1120) -> ("Stage1Temp"=w1115:i32, "Stage2Temp"=w1114:i32, "TcPressure"=w1113:i32)
                n538 = To Double Precision Float(number=w1115) -> (double precision float=w1112:dbl)
                n539 = To Double Precision Float(number=w1114) -> (double precision float=w1111:dbl)
                n540 = To Double Precision Float(number=w1113) -> (double precision float=w1110:dbl)
                n541 = Build Array(w1111) -> (w1108:dbl[])
                n542 = Build Array(w1110) -> (w1109:dbl[])
                n543 = Build Array(w1112) -> (w1107:dbl[])
                n544 = Bundle(cluster=w1116, "Cryopump Stage 1 Temp"=w1107, "Cryopump Stage 2 Temp"=w1108, "Compressor Temp"=w1109) -> (w1117:T8)
              }
              frame "Buffer Needs to be list" {
                n545 = One Button Dialog(message=w1121) -> ()  [unwired: 1 in, 1 out]
              }
            }
          }
        }
        n546 = Bundle By Name(cluster=w1094, "PumpTemps"=w1092) -> (w1099:T6)
      }
      frame "getZones" {
        w1130 = cluster{"ZoneSetPoint":dbl[], "ZoneTemp":dbl[]} {"ZoneSetPoint"=[], "ZoneTemp"=[]}
        n547 = Unbundle By Name(w1134) -> ("Http session"=w1138:T5, "URL prefex"=w1131:string)
        n548 = local read "Local Debug"() -> (w1132:bool)
        n549 = Flatten To JSON(anything=w1130) -> (JSON string=w1135:string)  [unwired: 2 in, 1 out]
        n550 = Concatenate Strings(w1131, "getZoneTemps" ("url")) -> (w1137:string)
        n551 = case shown="True" w1132 {
          tunnel: [w1167 w1168] -> _
          tunnel: [w1166 w1169] -> _
          tunnel: w1138 -> [_ _]
          tunnel: w1137 -> [w1165 w1172]
          tunnel: [w1164 w1170] -> w1133
          tunnel: [w1163 w1171] -> _
          tunnel: w1135 -> [_ w1173]
          frame False {
            n552 = call <vilib>:"GET.vi"("url"=w1165) -> ("client handle out"=w1166:T5, "headers"=w1163:string, "body"=w1164:string, "error out"=w1167:errorcluster)  [unwired: 11 in]
          }
          frame True {
            n553 = call-poly <vilib>:"POST.vi"("url"=w1172, "buffer"=w1173) -> ("client handle out"=w1169:T5, "headers"=w1171:string, "body"=w1170:string, "error out"=w1168:errorcluster)  [unwired: 10 in]
          }
        }
        n554 = Unflatten From JSON(JSON string=w1133, type and defaults=w1130) -> (value=w1129:cluster{"ZoneSetPoint":dbl[], "ZoneTemp":dbl[]})  [unwired: 5 in, 1 out]
        n555 = Unbundle By Name(w1129) -> ("ZoneSetPoint"=w1123:dbl[], "ZoneTemp"=w1125:dbl[])
        n556 = Initialize Array(0.0 ("element"), 18 ("dimension size")) -> (w1126:dbl[])
        n557 = for {
          N: 18 -> [_]
          tunnel: w1125 -> [w1142]
          shift-right: [w1141] -> w1122
          shift-left: w1126 -> [w1146]
          tunnel: w1123 -> [w1143]
          i -> [w1145]
          n558 = Quotient & Remainder(x=w1145, y=2) -> (x-y*floor(x/y)=w1144:i32)  [unwired: 1 out]
          n559 = Equal To 0?(x=w1144) -> (x = 0?=w1147:bool)
          n560 = case shown="False" w1147 {
            tunnel: w1146 -> [w1155 w1162]
            tunnel: w1145 -> [w1150 w1159]
            tunnel: [w1154 w1161] -> w1141
            tunnel: w1143 -> [w1151 _]
            tunnel: w1142 -> [_ w1160]
            frame False {
              n561 = Quotient & Remainder(x=w1150, y=2) -> (floor(x/y)=w1152:i32)  [unwired: 1 out]
              n562 = Index Array(array=w1151, index=w1152) -> (element=w1149:dbl)
              n563 = Replace Array Subset(array=w1155, new element=w1149, index=w1150) -> (w1154:dbl[])
            }
            frame True {
              n564 = Quotient & Remainder(x=w1159, y=2) -> (floor(x/y)=w1157:i32)  [unwired: 1 out]
              n565 = Index Array(array=w1160, index=w1157) -> (element=w1156:dbl)
              n566 = Replace Array Subset(array=w1162, new element=w1156, index=w1159) -> (w1161:dbl[])
            }
          }
        }
        n567 = Bundle By Name(cluster=w1134, "Zones"=w1122) -> (w1139:T6)
      }
      frame "masterDatabase" {
        n568 = Unbundle By Name(w1185) -> ("Thermocouples"=w1186:T3, "Pressure"=w1177:dbl[], "PumpTemps"=w1181:T4, "NumberTCs"=w1187:i32, "Zones"=w1174:dbl[])  [unwired: 1 out]
        n569 = Initialize Array(0.0 ("element"), w1187) -> (w1189:dbl[])
        n570 = Unbundle(w1181) -> ("Cp Stage 1 Temp"=w1180:dbl[], "Cp Stage 2 Temp"=w1179:dbl[], "Compressor Temp"=w1178:dbl[])
        n571 = Build Array (concatenate)(w1180, w1179, w1178) -> (w1176:dbl[])
        n572 = for {
          N: w1187 -> [_]
          shift-right: [w1199] -> w1175
          shift-left: w1189 -> [w1200]
          tunnel: w1186 -> [w1195]
          i -> [w1197]
          n573 = Quotient & Remainder(x=w1197, y=4) -> (x-y*floor(x/y)=w1194:i32, floor(x/y)=w1196:i32)
          n574 = Index Array(array=w1195, index (row)=w1196, index (col)=w1194) -> (element=w1193:T7)
          n575 = Unbundle By Name(w1193) -> ("Temperature"=w1192:string)
          n576 = Fract/Exp String To Number(string=w1192) -> (number=w1191:dbl)  [unwired: 3 in, 1 out]
          n577 = To Double Precision Float(number=w1191) -> (double precision float=w1201:dbl)
          n578 = Replace Array Subset(array=w1200, new element=w1201, index=w1197) -> (w1199:dbl[])
        }
        n579 = Build Array (concatenate)(dbl[] [0.0], w1177, w1174, w1175, w1176) -> (w1183:dbl[])
        n580 = Bundle By Name(cluster=w1185, "Database"=w1183) -> (w1184:T6)
      }
      frame "multipleGraphs" {
        n581 = local read "Custom Graph Selector"() -> (w1202:i32)
        n582 = for {
          N: 6 ("Numeric") -> [_]
          tunnel: w1205 -> [w1219]
          tunnel: w1204 -> [w1218]
          tunnel: w1202 -> [w1209]
          i -> [w1206]
          n583 = case shown="2" w1206 {
            tunnel: [w1265 w1266 w1268 w1270 w1272 w1274] -> w1211
            tunnel: [w1264 w1267 w1269 w1271 w1273 w1275] -> w1210
            frame 0, Default {
              n584 = control-ref of="Custom Chart 1 Selection"() -> (w1264:refnum<vi>)
              n585 = control-ref of="Custom Chart 1"() -> (w1265:refnum<vi>)
            }
            frame 1 {
              n586 = control-ref of="Custom Chart 2 Selection"() -> (w1267:refnum<vi>)
              n587 = control-ref of="Custom Chart 2"() -> (w1266:refnum<vi>)
            }
            frame 2 {
              n588 = control-ref of="Custom Chart 3 Selection"() -> (w1269:refnum<vi>)
              n589 = control-ref of="Custom Chart 3"() -> (w1268:refnum<vi>)
            }
            frame 3 {
              n590 = control-ref of="Custom Chart 4 Selection"() -> (w1271:refnum<vi>)
              n591 = control-ref of="Custom Chart 4"() -> (w1270:refnum<vi>)
            }
            frame 4 {
              n592 = control-ref of="Custom Chart 5 Selection"() -> (w1273:refnum<vi>)
              n593 = control-ref of="Custom Chart 5"() -> (w1272:refnum<vi>)
            }
            frame 5 {
              n594 = control-ref of="Custom Chart 6 Selection"() -> (w1275:refnum<vi>)
              n595 = control-ref of="Custom Chart 6"() -> (w1274:refnum<vi>)
            }
          }
          n596 = Equal?(x=w1209, y=w1206) -> (x = y?=w1207:bool)
          n597 = Unbundle By Name(w1218) -> ("Database"=w1216:dbl[], "numSensors"=w1217:i32)
          n598 = case shown="True" w1207 {
            tunnel: w1219 -> [_ w1233]
            tunnel: [w1222 w1227] -> w1215
            tunnel: [1000 w1226] -> w1214
            tunnel: w1210 -> [w1223 w1225]
            tunnel: [FALSE w1224] -> w1208
            frame False {
              n599 = property on="Property Node" class="LstBox (strict)"(reference=w1223) -> ("Item Symbols"=w1222:i32[])  [unwired: 1 in, 2 out]
            }
            frame True {
              n600 = property on="Property Node" class="LstBox (strict)"(reference=w1225) -> ("Item Symbols"=w1227:i32[])  [unwired: 1 in, 2 out]
              n601 = Decimal String To Number(string=w1233) -> (number=w1226:i32)  [unwired: 2 in, 1 out]
              n602 = Index Array(array=w1227, index=0) -> (element=w1228:i32)
              n603 = Equal?(x=37, y=w1228) -> (x = y?=w1230:bool)
              n604 = Equal To 0?(x=w1226) -> (x = 0?=w1232:bool)
              n605 = And(x=w1230, y=w1232) -> (x .and. y?=w1224:bool)
            }
          }
          n606 = case shown="False" w1208 {
            tunnel: [0 ("index") w1328] -> w1213
            tunnel: w1217 -> [w1282 w1324]
            tunnel: w1216 -> [w1281 _]
            tunnel: [w1280 _] -> w1212
            tunnel: w1214 -> [w1278 w1328]
            tunnel: w1215 -> [w1279 w1327]
            tunnel: w1210 -> [w1277 w1323]
            tunnel: w1211 -> [w1276 w1322]
            frame False {
              n607 = for {
                N: w1282 -> [_]
                tunnel: [w1301] -> w1280 mode=indexing
                tunnel: w1278 -> [w1295]
                tunnel: w1279 -> [w1290]
                tunnel: w1281 -> [w1287] mode=indexing
                tunnel: w1277 -> [w1285]
                tunnel: w1276 -> [w1284]
                i -> [w1288]
                n608 = Wait (ms)(milliseconds to wait=u32 0) -> ()  [unwired: 1 out]
                n609 = Get Date/Time In Seconds() -> (seconds since 1Jan1904=w1303:timestamp)
                n610 = Bundle By Name("t0"=w1303) -> (w1302:waveform(dbl))  [unwired: 1 in]
                n611 = Build Array(w1287) -> (w1286:dbl[])
                n612 = Bundle By Name(cluster=w1302, "Y"=w1286) -> (w1301:waveform(dbl))
                n613 = Index Array(array=w1290, index=w1295) -> (element=w1293:i32)
                n614 = Index Array(array=w1290, index=w1295) -> (element=w1296:i32)
                n615 = Equal?(x=w1293, y=38) -> (x = y?=w1292:bool)
                n616 = Equal?(x=w1296, y=37) -> (x = y?=w1298:bool)
                n617 = Equal?(x=w1288, y=w1295) -> (x = y?=w1291:bool)
                n618 = And(x=w1291, y=w1292) -> (x .and. y?=w1289:bool)
                n619 = And(x=w1291, y=w1298) -> (x .and. y?=w1297:bool)
                n620 = case shown="True" w1297 {
                  tunnel: w1290 -> [_ w1321]
                  tunnel: w1295 -> [_ _]
                  tunnel: w1288 -> [_ w1316]
                  tunnel: w1284 -> [_ w1313]
                  tunnel: w1285 -> [_ w1314]
                  frame False {
                  }
                  frame True {
                    n621 = property on="Property Node" class="WFChart (strict)"(reference=w1313, "Active Plot"=w1316) -> (reference out=w1319:refnum<vi>)  [unwired: 1 in, 1 out]
                    n622 = Replace Array Subset(array=w1321, new element=38, index=w1316) -> (w1317:i32[])
                    n623 = property on="Property Node" class="WFChart (strict)"(reference=w1313) -> ("Plot.Plot Color"=w1315:u32)  [unwired: 1 in, 2 out]
                    n624 = property on="Property Node" class="WFChart (strict)"(reference=w1319, "Plot.Visible?"=TRUE ("Plot.Visible")) -> ()  [unwired: 1 in, 2 out]
                    n625 = property on="Property Node" class="LstBox (strict)"(reference=w1314, "Active Row"=w1316) -> ()  [unwired: 1 in, 2 out]
                    n626 = property on="Property Node" class="LstBox (strict)"(reference=w1314, "CellBG"=w1315) -> ()  [unwired: 1 in, 2 out]
                    n627 = property on="Property Node" class="LstBox (strict)"(reference=w1314, "Item Symbols"=w1317) -> ()  [unwired: 1 in, 2 out]
                  }
                }
                n628 = case shown="True" w1289 {
                  tunnel: w1290 -> [_ w1312]
                  tunnel: w1288 -> [_ w1305]
                  tunnel: w1284 -> [_ w1306]
                  tunnel: w1285 -> [_ w1307]
                  frame False {
                  }
                  frame True {
                    n629 = property on="Property Node" class="WFChart (strict)"(reference=w1306, "Active Plot"=w1305) -> (reference out=w1310:refnum<vi>)  [unwired: 1 in, 1 out]
                    n630 = Replace Array Subset(array=w1312, new element=37, index=w1305) -> (w1308:i32[])
                    n631 = property on="Property Node" class="WFChart (strict)"(reference=w1310, "Plot.Visible?"=FALSE ("Plot.Visible")) -> ()  [unwired: 1 in, 2 out]
                    n632 = property on="Property Node" class="LstBox (strict)"(reference=w1307, "Active Row"=w1305) -> ()  [unwired: 1 in, 2 out]
                    n633 = property on="Property Node" class="LstBox (strict)"(reference=w1307, "CellBG"=u32 13816530 ("Active Row:Cell Background Color")) -> ()  [unwired: 1 in, 2 out]
                    n634 = property on="Property Node" class="LstBox (strict)"(reference=w1307, "Item Symbols"=w1308) -> ()  [unwired: 1 in, 2 out]
                  }
                }
              }
            }
            frame True {
              n635 = for {
                N: w1324 -> [_]
                tunnel: w1327 -> [_]
                tunnel: w1323 -> [w1330]
                tunnel: w1322 -> [w1329]
                i -> [w1331]
                n636 = property on="Property Node" class="WFChart (strict)"(reference=w1329, "Active Plot"=w1331) -> (reference out=w1334:refnum<vi>)  [unwired: 1 in, 1 out]
                n637 = property on="Property Node" class="WFChart (strict)"(reference=w1334, "Plot.Visible?"=FALSE ("Plot.Visible")) -> ()  [unwired: 1 in, 2 out]
                n638 = property on="Property Node" class="LstBox (strict)"(reference=w1330, "Active Row"=w1331) -> ()  [unwired: 1 in, 2 out]
                n639 = property on="Property Node" class="LstBox (strict)"(reference=w1330, "CellBG"=u32 13816530 ("Active Row:Cell Background Color")) -> ()  [unwired: 1 in, 2 out]
              }
              n640 = Initialize Array(37, w1324) -> (w1325:i32[])
              n641 = property on="Property Node" class="LstBox (strict)"(reference=w1323, "Item Symbols"=w1325) -> ()  [unwired: 1 in, 2 out]
            }
          }
          n642 = case shown="5" w1206 {
            tunnel: w1213 -> [w1235 w1240 w1245 w1250 w1255 w1260]
            tunnel: w1212 -> [w1234 w1239 w1244 w1249 w1254 w1259]
            frame 0, Default {
              n643 = Build Array (concatenate)(waveform(dbl) {"t0"=timestamp(0 s since 1904-01-01), "dt"=1.0, "Y"=[]} ("element"), w1234) -> (w1238:waveform(dbl)[])
              n644 = Delete From Array(array=w1238, index=w1235) -> (array with subset deleted=→"Custom Chart 1":waveform(dbl)[])  [unwired: 1 in, 1 out]
            }
            frame 1 {
              n645 = Build Array (concatenate)(waveform(dbl) {"t0"=timestamp(0 s since 1904-01-01), "dt"=1.0, "Y"=[]} ("element"), w1239) -> (w1243:waveform(dbl)[])
              n646 = Delete From Array(array=w1243, index=w1240) -> (array with subset deleted=→"Custom Chart 2":waveform(dbl)[])  [unwired: 1 in, 1 out]
            }
            frame 2 {
              n647 = Build Array (concatenate)(waveform(dbl) {"t0"=timestamp(0 s since 1904-01-01), "dt"=1.0, "Y"=[]} ("element"), w1244) -> (w1248:waveform(dbl)[])
              n648 = Delete From Array(array=w1248, index=w1245) -> (array with subset deleted=→"Custom Chart 3":waveform(dbl)[])  [unwired: 1 in, 1 out]
            }
            frame 3 {
              n649 = Build Array (concatenate)(waveform(dbl) {"t0"=timestamp(0 s since 1904-01-01), "dt"=1.0, "Y"=[]} ("element"), w1249) -> (w1253:waveform(dbl)[])
              n650 = Delete From Array(array=w1253, index=w1250) -> (array with subset deleted=→"Custom Chart 4":waveform(dbl)[])  [unwired: 1 in, 1 out]
            }
            frame 4 {
              n651 = Build Array (concatenate)(waveform(dbl) {"t0"=timestamp(0 s since 1904-01-01), "dt"=1.0, "Y"=[]} ("element"), w1254) -> (w1258:waveform(dbl)[])
              n652 = Delete From Array(array=w1258, index=w1255) -> (array with subset deleted=→"Custom Chart 5":waveform(dbl)[])  [unwired: 1 in, 1 out]
            }
            frame 5 {
              n653 = Build Array (concatenate)(waveform(dbl) {"t0"=timestamp(0 s since 1904-01-01), "dt"=1.0, "Y"=[]} ("element"), w1259) -> (w1263:waveform(dbl)[])
              n654 = Delete From Array(array=w1263, index=w1260) -> (array with subset deleted=→"Custom Chart 6":waveform(dbl)[])  [unwired: 1 in, 1 out]
            }
          }
        }
      }
      frame "setThermalProfile" {
        n655 = event shown="[0] \"Set Z 1\": Mouse Down" {
          selector: _ -> [_]
          dyn-events: _ -> [_]
          timeout: _ -> [_]
          tunnel: T2 {"profiles"=[]} -> [w1344]
          event "Set Z 1": Mouse Down {
            n656 = event-data() -> ()  [unwired: 1 in, 8 out]
            n657 = local read "Cluster"() -> (w1338:T2)
            n658 = Unbundle By Name(w1338) -> ("profiles"=w1339:T16)
            n659 = Array To Cluster(array=w1339) -> (cluster=w1343:T17)
            n660 = local read "Zone 1 Temp"() -> (w1341:u16)
            n661 = Unbundle By Name(w1343) -> ("profiles[0]"=w1342:T1)
            n662 = Bundle By Name(cluster=w1342, "zone"=1, "average"=w1341) -> (→"output cluster":T1)
            "Cluster" <- w1344
          }
        }
      }
      frame "exit" {
        n663 = Unbundle By Name(w1346) -> ("Http session"=w1347:T5)
        n664 = call <vilib>:"CloseHandle.vi"("client handle"=w1347, "error in (no error)"=w1349) -> ("error out"=w1348:errorcluster)  [unwired: 13 in]
        n665 = Bundle By Name(cluster=w1346, "go"=FALSE ("Bundle Element")) -> (w1350:T6)
      }
      frame Default {
        n666 = call "Unknown Message Dialog.vi"("error in (no error)"=w1353, "event name"=w1352) -> ("error out"=w1351:errorcluster)  [unwired: 9 in]
      }
    }
    n667 = Unbundle By Name(w29) -> ("go"=w28:bool)
    n668 = call "log system event.vi"("error in (no error)"=w31) -> ("error out"=w30:errorcluster)  [unwired: 9 in, 1 out]
  }
  n669 = call "Unload Module.vi"("error in (no error)"=w8) -> ()  [unwired: 10 in, 1 out]
  n670 = property on="Waveform Chart" class="WFChart (strict)" props=["Plot", "Visible?"]() -> ()  [unwired: 2 in, 3 out]
